vi "3D_Plotter_MATLAB.vi"(1 "Job Directory":path) -> (2 "Saved Automatically?":bool, 3 "gnuplotScript":string, 4 "Plot data file":path)   [LabVIEW 2022 SP3]
uses:
  Controls/Global_mode.ctl
  Data plotting/MATLAB/MATLAB_Mode.ctl
  <vilib>/Utility/error.llb/Trim Whitespace One-Sided.vi
  Results_plotter_Global.vi
  Globals/Constants_global.vi
  Data plotting/subVIs/Plot_Values_Global.vi
  <vilib>/Analysis/NI_AALBase.lvlib
panel:
  out "Output file":path
  out "Plot Folder":string[](array[string])
  out "Duplicate Plot":bool
  out "Selectors":i32[](array[numeric])
  out "stl filenames":string[][](array[string])
  out "Max Min array":dbl[][][][](array[numeric])
  out "stl Files":string[](array[string])
  out "stl Limits":sgl[][](array[numeric])
  out "C Limits":cluster{dbl[]}[](array[cluster])
  out "ldListDatafileShown":string[](array[string])
  out "Last Plot Index":i32[](array[numeric])
  out "Z per Figure":dbl[][](array[numeric])
  out "Y per Figure":dbl[][](array[numeric])
  out "X per Figure":dbl[][](array[numeric])
  out "All Z":dbl[](array[numeric])
  out "All Y":dbl[](array[numeric])
  out "All X":dbl[](array[numeric])
  out "Plot Titles":string[](array[string])
  out "Number of Figures":i32
  out "Plot":i32[][](array[numeric])
  out "X Labels":bool[](array[boolean])
  out "Y labels":bool[](array[boolean])
  in  "Tab Control":T1(tab)
  in  "Show Save Option?":bool
  in  "Font Size":string="10"
  in  "Height":string="0.02"
  in  "Width":string="0.2"
  in  "BottomEdge":string="0.05"
  in  "LeftEdge":string="0.4"
  in  "MainTitleFontSize":string="12"
  in  "Vectors":bool
  in  "Streamlines":bool
  in  "W Vector":u16(ring) items=["None", "Date of Measurement", "Time Measurement Commenced", "QA Code", "File", "Subproject", "Model Scale", "Hav (m)", "Spire Size", "Meas Instru Type", "Profile Type", "Ref Velocity (m/s)", "Uh_Uref Ratio", "Uref (m/s)", "Source Flow Rate (l/min)", "Stability", "Wind Direction (Deg)", "Wind Direction", "Magic Case", "Roughness Layout", "Turntable Size", "X (m) fs", "Y (m) fs", "Z (m) fs", "Z/Hav", "Legend1", "Legend2", "Legend3", "LegendDose", "Source", "X Pos (mm)", "Y Pos (mm)", "Z Pos (mm)", "Location XY fs", "U/Uref", "V/Uref", "W/Uref", "Wind speed/Uref", "u^2/Uref^2", "v^2/Uref^2", "w^2/Uref^2", "uv/Uref^2", "uw/Uref^2", "U (m/s)", "V (m/s)", "W (m/s)", "u^2 (m/s)^2", "v^2 (m/s)^2", "w^2 (m/s)^2", "uv (m/s)^2", "uw (m/s)^2", "U/Uref Std Error", "V/Uref Std Error", "W/Uref Std Error", "u^2/Uref^2 Std Error", "v^2/Uref^2 Std Error", "w^2/Uref^2 Std Error", "uv/Uref^2 Std Error", "uw/Uref^2 Std Error", "U (m/s) Std Error", "V (m/s) Std Error", "W (m/s) Std Error", "u^2 (m/s)^2 Std Error", "v^2 (m/s)^2 Std Error", "w^2 (m/s)^2 Std Error", "uv (m/s)^2 Std Error", "uw (m/s)^2 Std Error", "Atmos Pressure (mBar)", "Lab Ref Temperature (Deg C)", "Meas Time (min)", "Current Filepath", "Raw Data Filename", "Template File Used", "EnFlo_Tunnel Trav1 Pos Z", "EnFlo_Tunnel Trav1 Pos Y", "EnFlo_Tunnel Trav1 Pos X", "Coordinate System", "Original Results Filename", "Legend5", "Av LDA Sampling Rate", "Legend6", "Legend7", "K2", "Bldg12", "EnFlo_Tunnel Metadata Bldg12", "Current File 2nd Folder level"]
  in  "U Vector":u16(ring) items=["None", "Date of Measurement", "Time Measurement Commenced", "QA Code", "File", "Subproject", "Model Scale", "Hav (m)", "Spire Size", "Meas Instru Type", "Profile Type", "Ref Velocity (m/s)", "Uh_Uref Ratio", "Uref (m/s)", "Source Flow Rate (l/min)", "Stability", "Wind Direction (Deg)", "Wind Direction", "Magic Case", "Roughness Layout", "Turntable Size", "X (m) fs", "Y (m) fs", "Z (m) fs", "Z/Hav", "Legend1", "Legend2", "Legend3", "LegendDose", "Source", "X Pos (mm)", "Y Pos (mm)", "Z Pos (mm)", "Location XY fs", "U/Uref", "V/Uref", "W/Uref", "Wind speed/Uref", "u^2/Uref^2", "v^2/Uref^2", "w^2/Uref^2", "uv/Uref^2", "uw/Uref^2", "U (m/s)", "V (m/s)", "W (m/s)", "u^2 (m/s)^2", "v^2 (m/s)^2", "w^2 (m/s)^2", "uv (m/s)^2", "uw (m/s)^2", "U/Uref Std Error", "V/Uref Std Error", "W/Uref Std Error", "u^2/Uref^2 Std Error", "v^2/Uref^2 Std Error", "w^2/Uref^2 Std Error", "uv/Uref^2 Std Error", "uw/Uref^2 Std Error", "U (m/s) Std Error", "V (m/s) Std Error", "W (m/s) Std Error", "u^2 (m/s)^2 Std Error", "v^2 (m/s)^2 Std Error", "w^2 (m/s)^2 Std Error", "uv (m/s)^2 Std Error", "uw (m/s)^2 Std Error", "Atmos Pressure (mBar)", "Lab Ref Temperature (Deg C)", "Meas Time (min)", "Current Filepath", "Raw Data Filename", "Template File Used", "EnFlo_Tunnel Trav1 Pos Z", "EnFlo_Tunnel Trav1 Pos Y", "EnFlo_Tunnel Trav1 Pos X", "Coordinate System", "Original Results Filename", "Legend5", "Av LDA Sampling Rate", "Legend6", "Legend7", "K2", "Bldg12", "EnFlo_Tunnel Metadata Bldg12", "Current File 2nd Folder level"]
  in  "V Vector":u16(ring) items=["None", "Date of Measurement", "Time Measurement Commenced", "QA Code", "File", "Subproject", "Model Scale", "Hav (m)", "Spire Size", "Meas Instru Type", "Profile Type", "Ref Velocity (m/s)", "Uh_Uref Ratio", "Uref (m/s)", "Source Flow Rate (l/min)", "Stability", "Wind Direction (Deg)", "Wind Direction", "Magic Case", "Roughness Layout", "Turntable Size", "X (m) fs", "Y (m) fs", "Z (m) fs", "Z/Hav", "Legend1", "Legend2", "Legend3", "LegendDose", "Source", "X Pos (mm)", "Y Pos (mm)", "Z Pos (mm)", "Location XY fs", "U/Uref", "V/Uref", "W/Uref", "Wind speed/Uref", "u^2/Uref^2", "v^2/Uref^2", "w^2/Uref^2", "uv/Uref^2", "uw/Uref^2", "U (m/s)", "V (m/s)", "W (m/s)", "u^2 (m/s)^2", "v^2 (m/s)^2", "w^2 (m/s)^2", "uv (m/s)^2", "uw (m/s)^2", "U/Uref Std Error", "V/Uref Std Error", "W/Uref Std Error", "u^2/Uref^2 Std Error", "v^2/Uref^2 Std Error", "w^2/Uref^2 Std Error", "uv/Uref^2 Std Error", "uw/Uref^2 Std Error", "U (m/s) Std Error", "V (m/s) Std Error", "W (m/s) Std Error", "u^2 (m/s)^2 Std Error", "v^2 (m/s)^2 Std Error", "w^2 (m/s)^2 Std Error", "uv (m/s)^2 Std Error", "uw (m/s)^2 Std Error", "Atmos Pressure (mBar)", "Lab Ref Temperature (Deg C)", "Meas Time (min)", "Current Filepath", "Raw Data Filename", "Template File Used", "EnFlo_Tunnel Trav1 Pos Z", "EnFlo_Tunnel Trav1 Pos Y", "EnFlo_Tunnel Trav1 Pos X", "Coordinate System", "Original Results Filename", "Legend5", "Av LDA Sampling Rate", "Legend6", "Legend7", "K2", "Bldg12", "EnFlo_Tunnel Metadata Bldg12", "Current File 2nd Folder level"]
  in  "Manual_stl file":bool
  in  "Show whole Stl file":bool=TRUE
  in  "Stl File":u16(ring) items=["", "StreetCanyonGeometry.stl"]
  in  "Z Limits Auto":bool=TRUE
  in  "Location Z limits":string="-2000;2000"
  out "Y Limit":string
  out "X Limit":string
  in  "Concentration?":bool
  in  "Range Auto":bool=TRUE
  in  "Same Location limits for all plots":bool=TRUE
  in  "Swop Series and Plots":bool
  in  "mSingleColorbar":bool=TRUE
  in  "Y Limits Auto":bool=TRUE
  in  "X Limits Auto":bool=TRUE
  in  "Location X limits":string="-2000;2000"
  in  "nRows":u8=3 min=1
  in  "nCols":u8=3 min=1
  in  "cScatterPointSize":string="5"
  in  "Plotting":enum8{"Lin", "Log"}(ring)
  in  "fvectorRotation":string="0;0;0"
  in  "cdColorbarRange":string="0.01;100"
  in  "No Of decades":i32=3 min=1 max=10
  in  "Location Y limits":string="-2000;2000"
  out "Z Limit":string
  in  "ViewAngles":string="-115;35"
  in  "Transparency":string="0.5"
  in  "Streamline Density":string="0.5"
  in  "Open in Acrobat":bool=TRUE
  in  "Show Channels with range of Values?":bool
  in  "Page Title Pre Block":string
  in  "Page Title Post Block":string
  in  "Values to include in Page Title":i32[](listbox)
  out "Final Title":string
  out "Plot Legends Auto":string[](array[string])
  out "No of Series supplied":i32
  out "AuditTrail":string[](array[string])
  out "Desired Legends":string[][](array[string])
  out "Table":string[][](table)
  # "Plot XY axes control"
  # "Color Bar"
  # "Overall Page Title"
  # "There are as many graphs as there are titles (from Selector 2)...."
  # "Plot Styles"
  # "Each graph contains plots from Selector 1..."
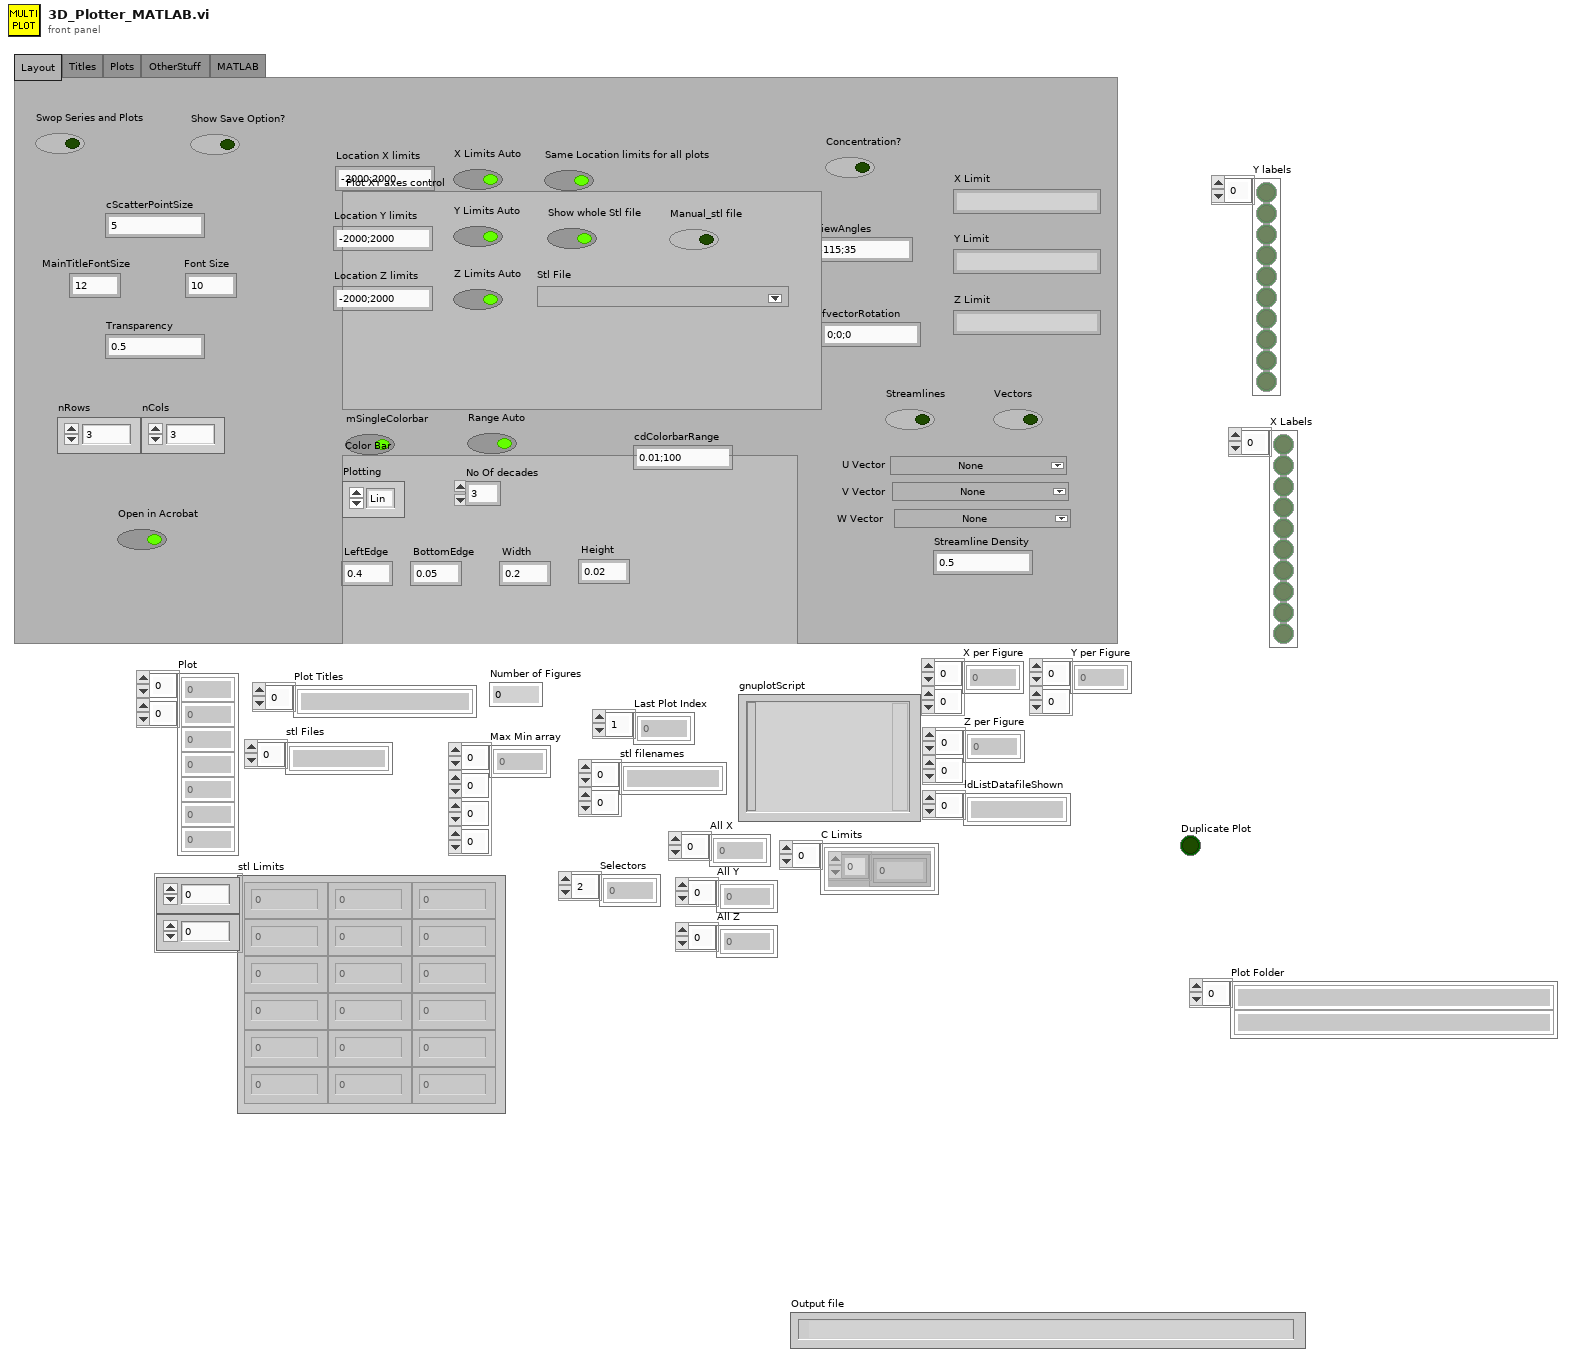
[diagram p1: front panel]
types:
  T1 = enum32{"Layout", "Titles", "Plots", "OtherStuff ", "MATLAB"}
  T2 = typedef "RFP_Plot_Metadata.ctl" = cluster{"Row Number":i32[], "Error Bars":T3, "X Label":string, "Y Label":string, "Blanks NaNs":i32[]}
  T3 = typedef "Error_bars_index.ctl" = cluster{"Upper":i32, "Lower":i32, "St Error":i32}
  T4 = typedef "Global_mode.ctl" = enum16{"Read Global", "Load Global From File", "Write Global to File"}
  T5 = typedef "MATLAB_Mode.ctl" = enum16{"1D Plotter", "2D Plotter", "LP Plotter", "7HP UVW"}
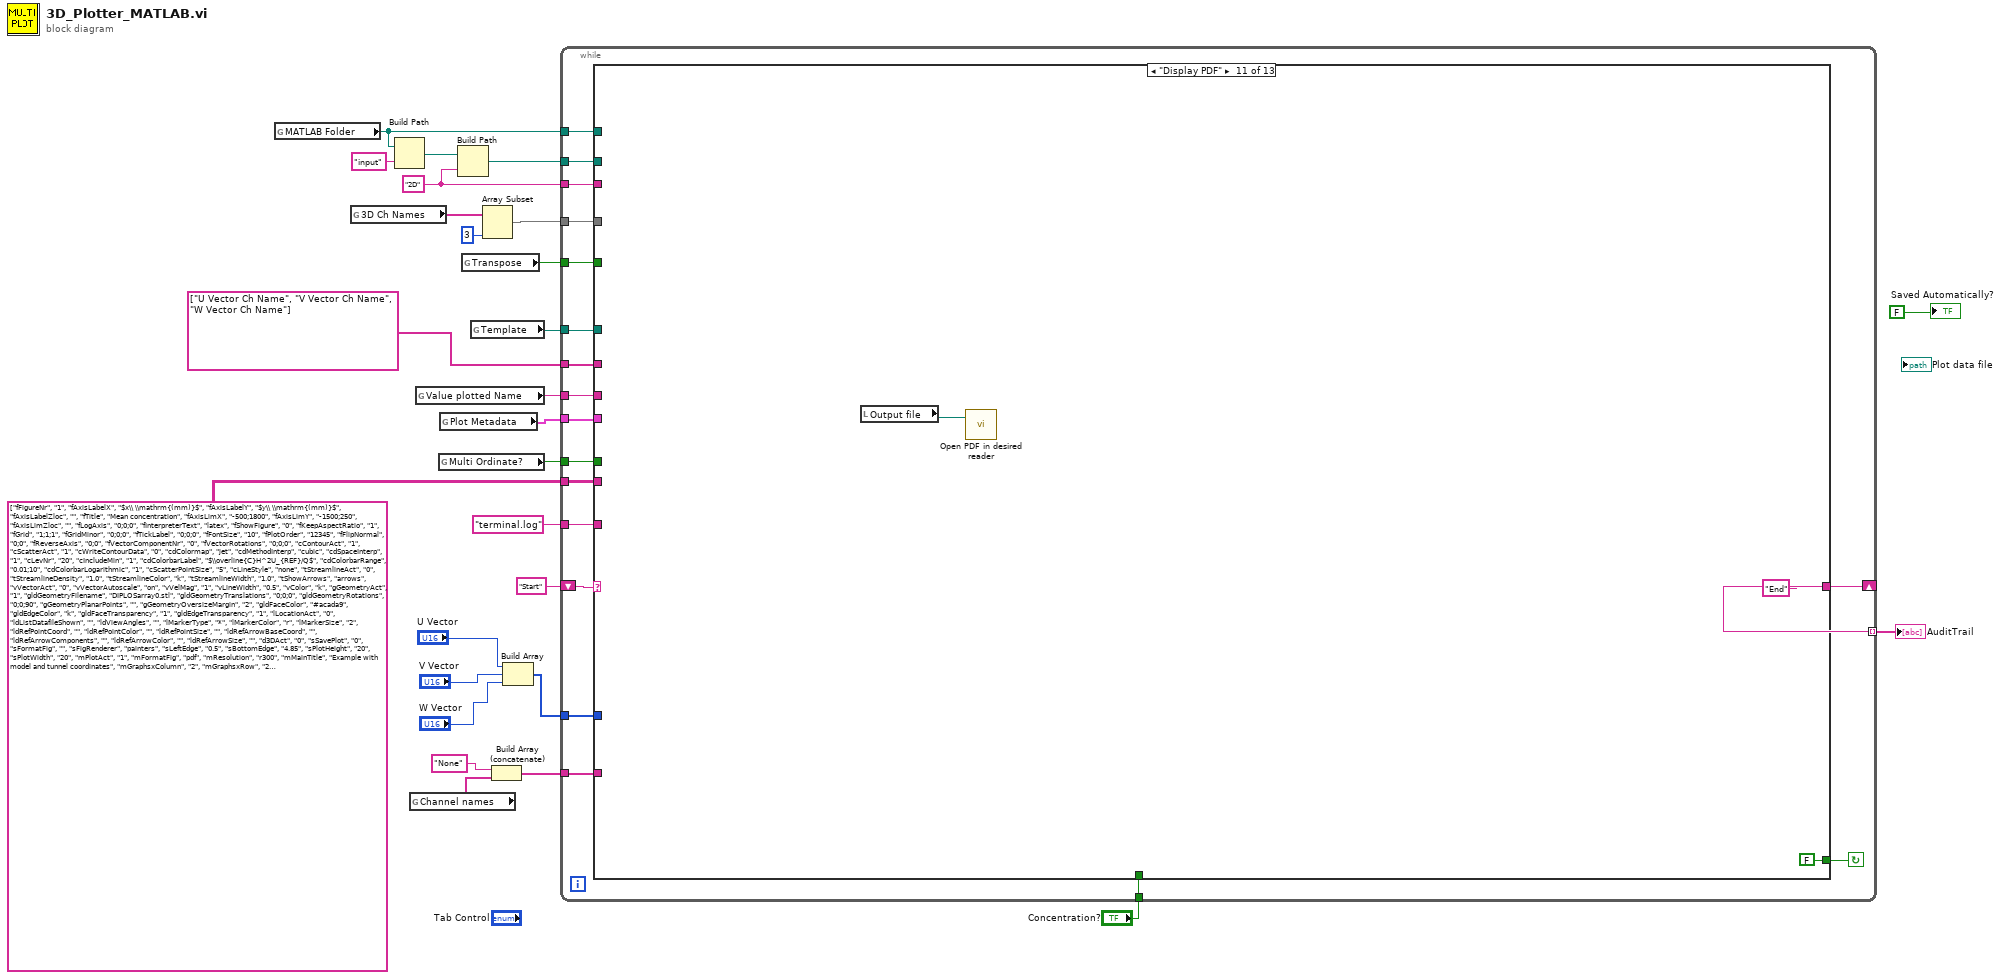
[diagram p0: block diagram]
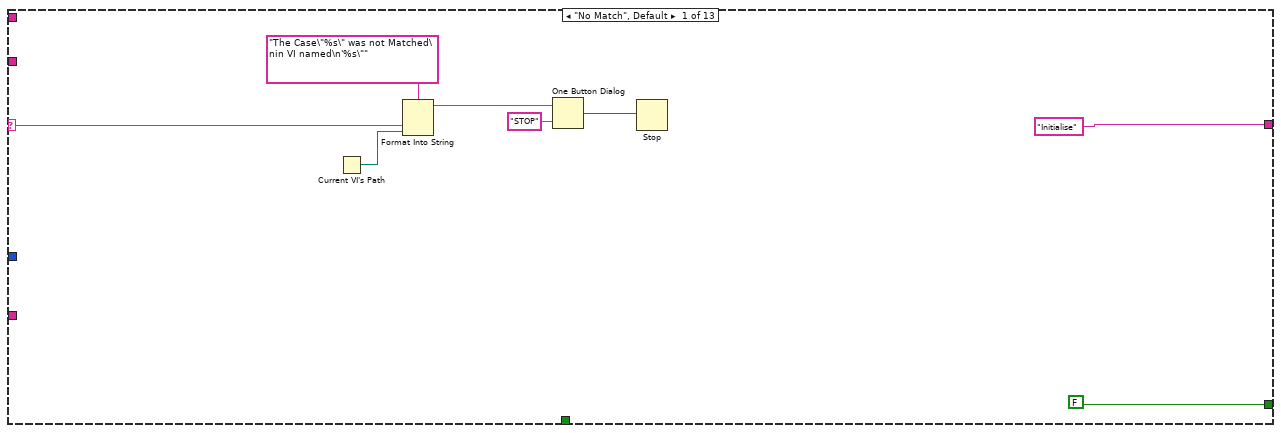
[diagram p2: hidden frame]
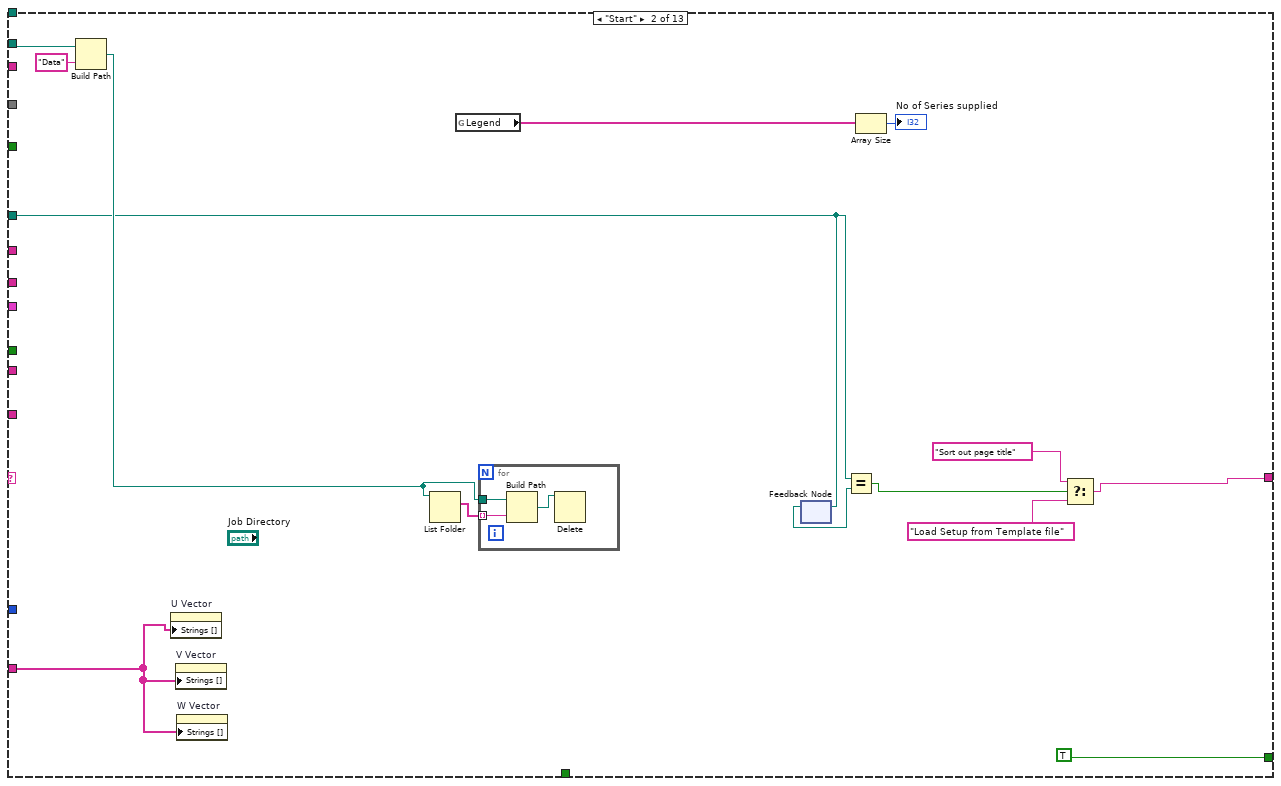
[diagram p3: hidden frame]
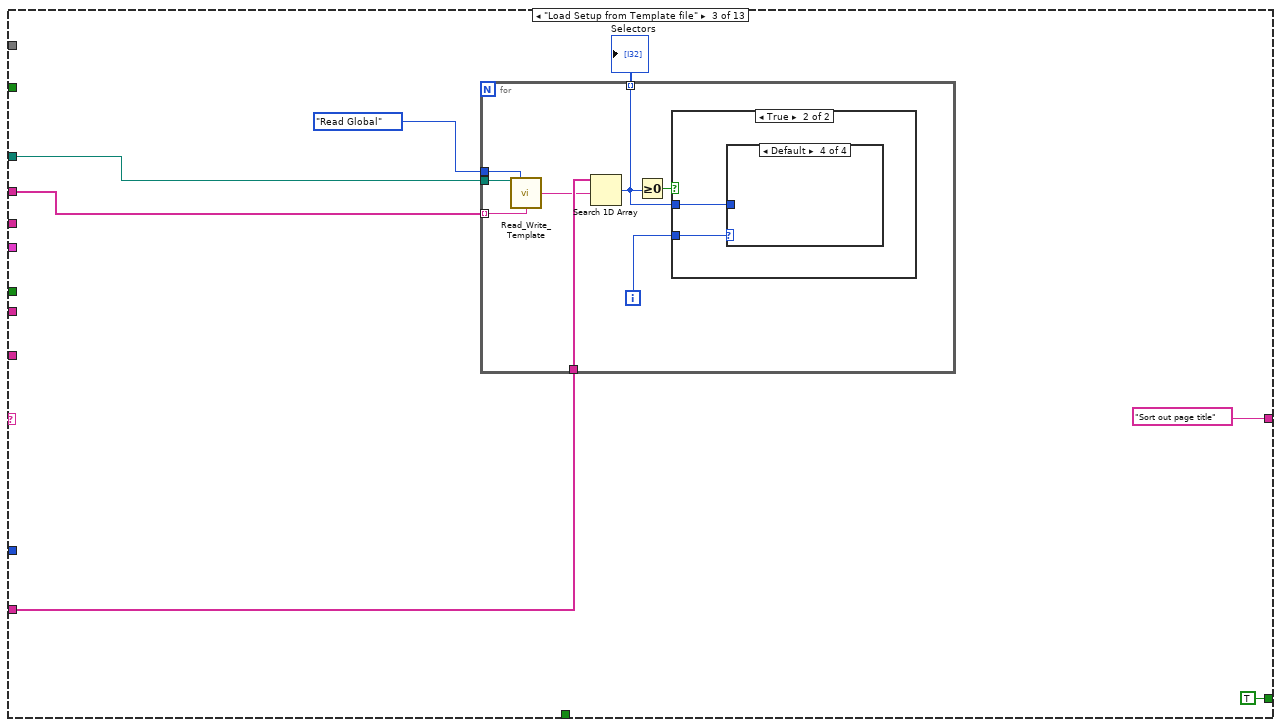
[diagram p4: hidden frame]
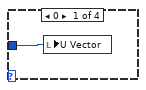
[diagram p6: hidden frame]
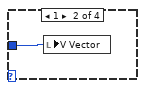
[diagram p7: hidden frame]
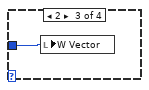
[diagram p8: hidden frame]
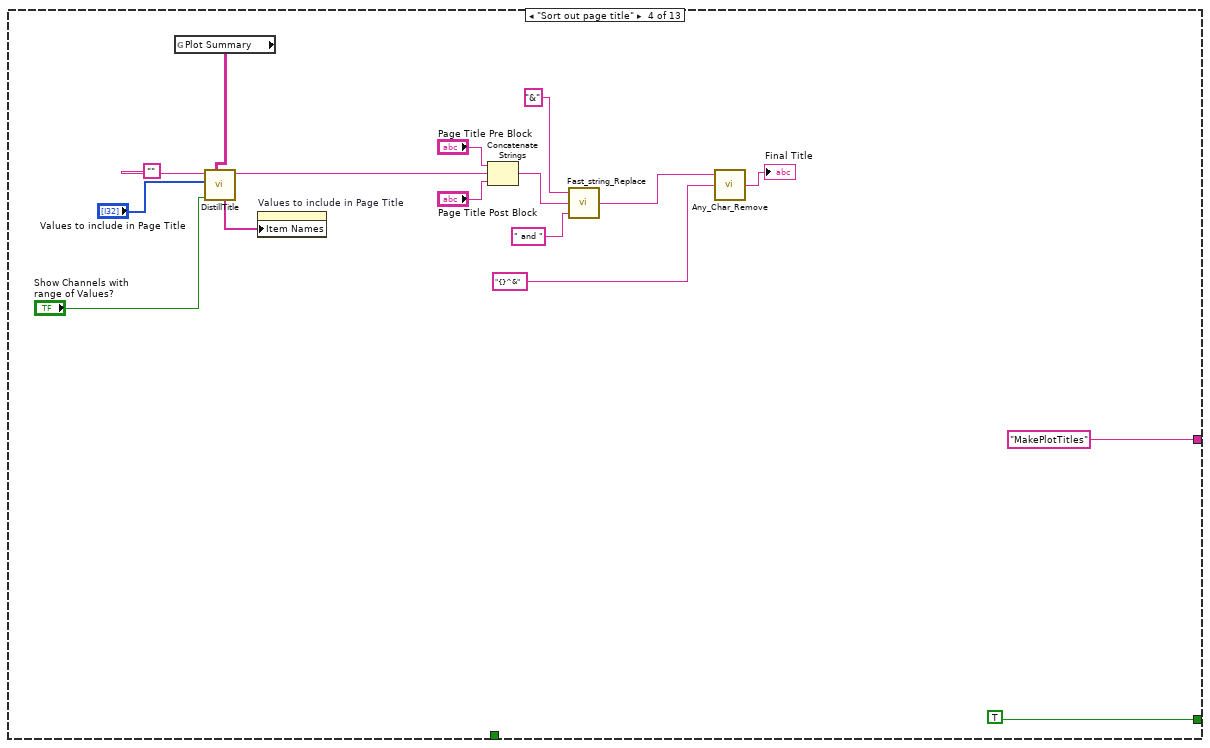
[diagram p9: hidden frame]
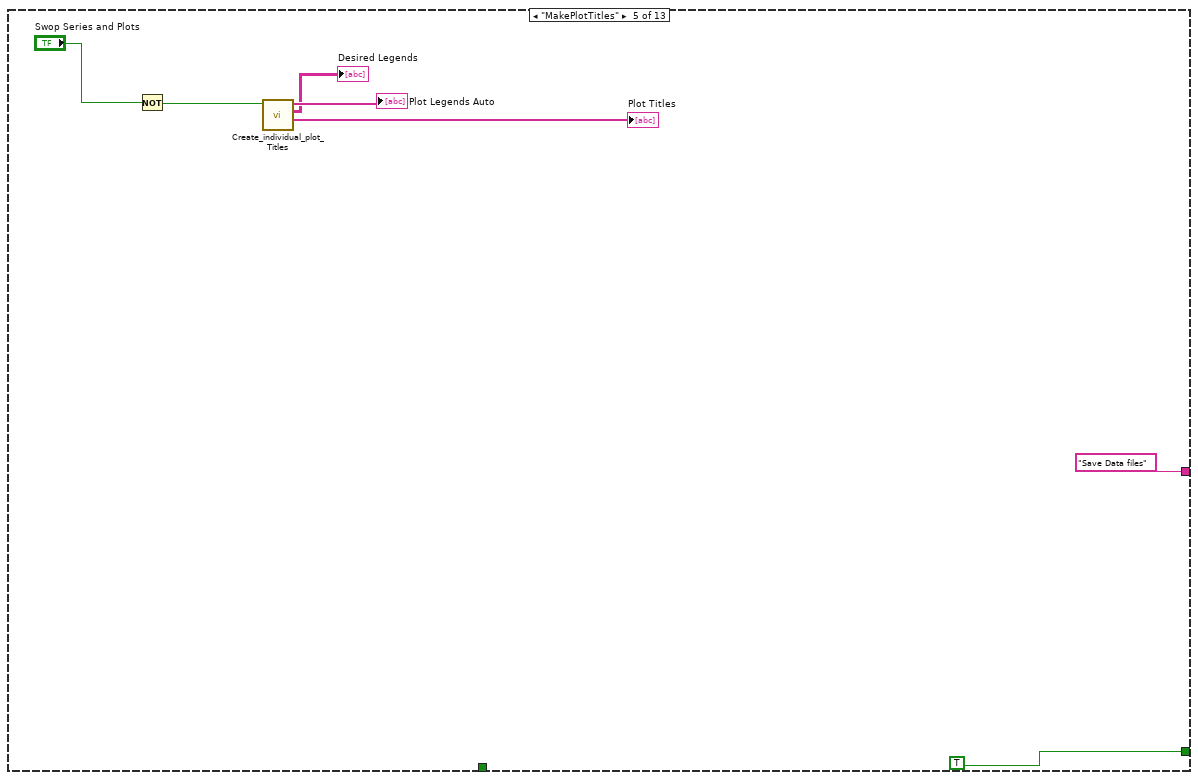
[diagram p10: hidden frame]
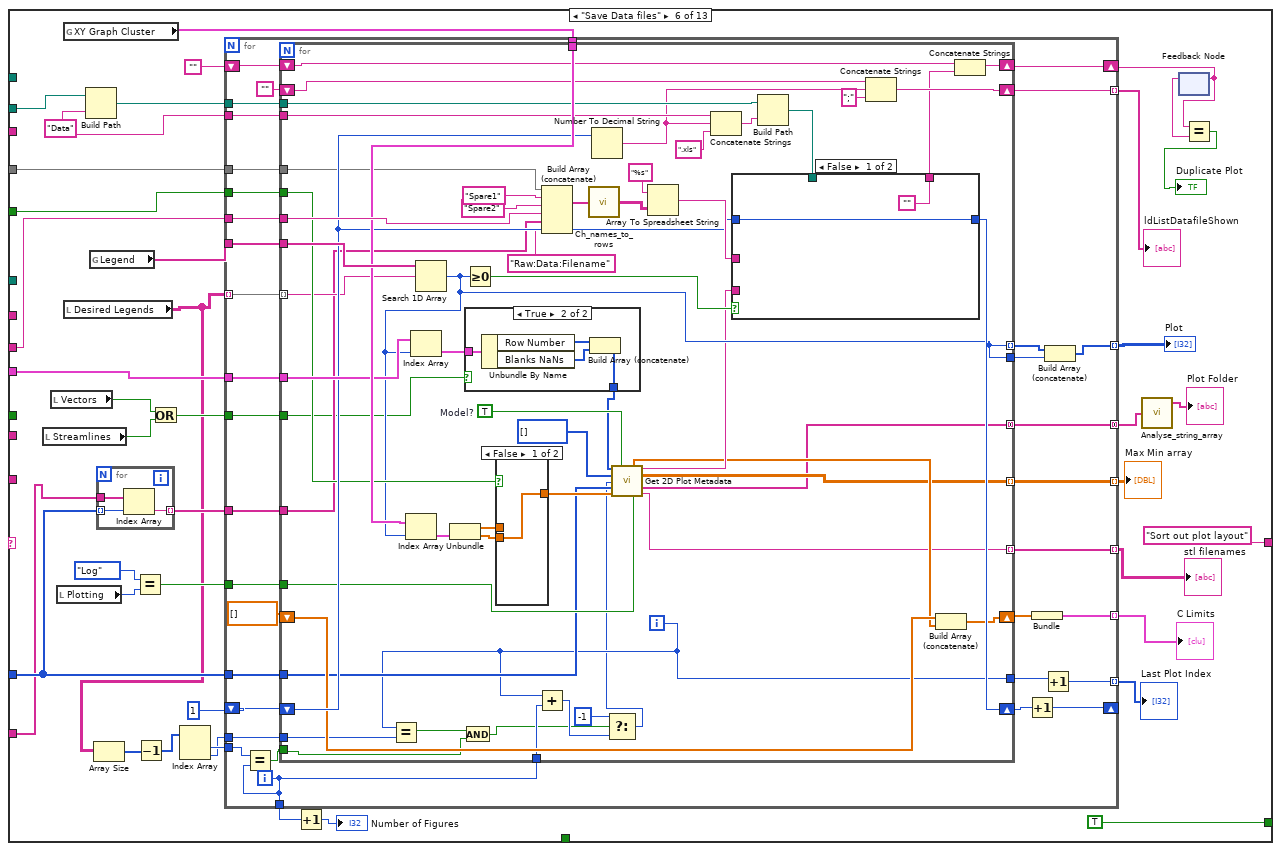
[diagram p11: hidden frame]
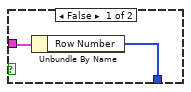
[diagram p12: hidden frame]
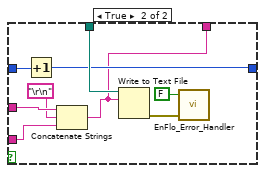
[diagram p14: hidden frame]
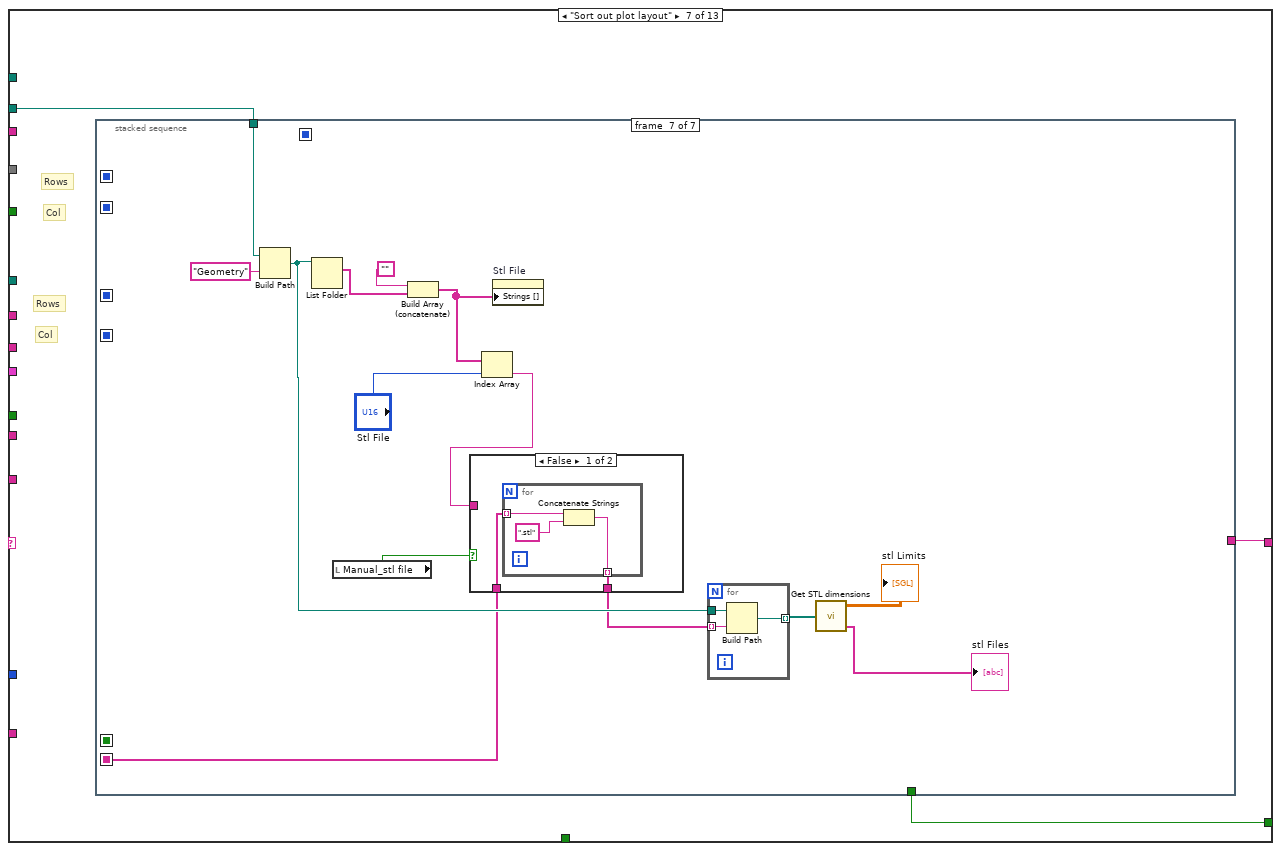
[diagram p15: hidden frame]
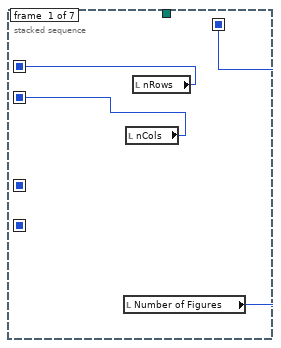
[diagram p16: hidden frame]
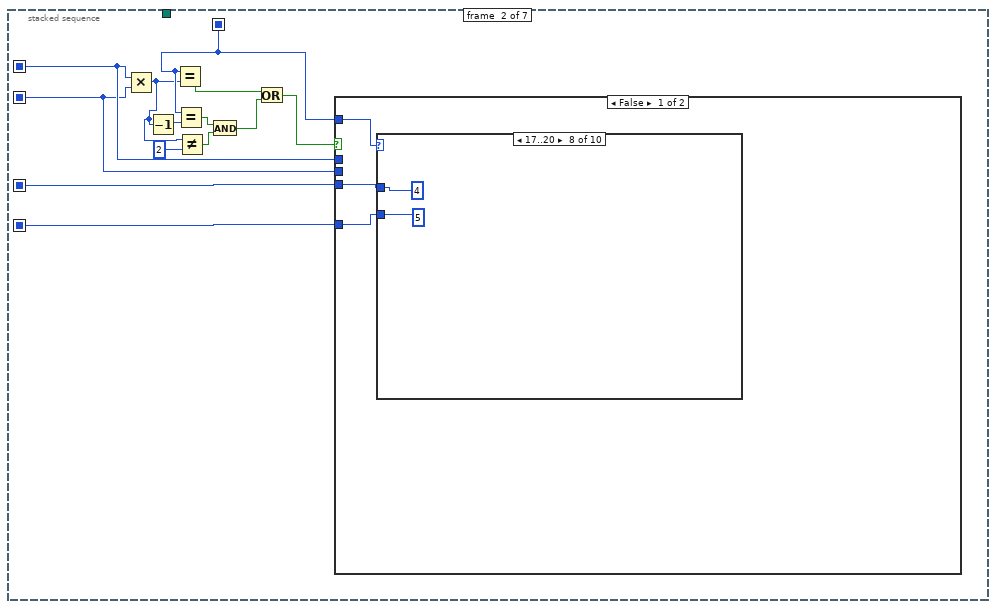
[diagram p17: hidden frame]
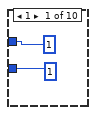
[diagram p18: hidden frame]
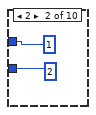
[diagram p19: hidden frame]
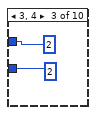
[diagram p20: hidden frame]
diagram:
  w1 = "2D" ("name or relative path")
  n1 = global read "Constants_global.vi" "MATLAB Folder"() -> (w2:path)
  n2 = global read "Results_plotter_Global.vi" "3D Ch Names"() -> (w13:string[])
  n3 = Build Path(base path=w2, name or relative path="input") -> (appended path=w19:path)
  n4 = global read "Results_plotter_Global.vi" "Channel names"() -> (w6:string[])
  n5 = global read "Results_plotter_Global.vi" "Value plotted Name"() -> (w26:string)
  n6 = global read "Results_plotter_Global.vi" "Multi Ordinate?"() -> (w22:bool)
  n7 = global read "Results_plotter_Global.vi" "Plot Metadata"() -> (w16:T2[])
  n8 = Build Path(base path=w19, name or relative path=w1) -> (appended path=w18:path)
  n9 = global read "Results_plotter_Global.vi" "Transpose"() -> (w23:bool)
  n10 = global read "Results_plotter_Global.vi" "Template"() -> (w4:path)
  n11 = Array Subset(array=w13, length=3) -> (w12:string[])  [unwired: 1 in]
  n12 = Build Array (concatenate)("None", w6) -> (w5:string[])
  n13 = Build Array("U Vector", "V Vector", "W Vector") -> (w8:u16[])
  n14 = while {
    shift-left: "Start" -> [w44]
    shift-right: [w39] -> _
    tunnel: w26 -> [w43]
    tunnel: "terminal.log" -> [w42]
    tunnel: w23 -> [w41]
    tunnel: w22 -> [w40]
    tunnel: [w39] -> w21 mode=indexing
    tunnel: w18 -> [w38]
    tunnel: string[][] [["fFigureNr", "1"], ["fAxisLabelX", "$x\\ \\mathrm{(mm)}$"], ["fAxisLabelY", "$y\\ \\mathrm{(mm)}$"], ["fAxisLabelZloc", ""], ["fTitle", "Mean concentration"], ["fAxisLimX", "-500;1800"], ["fAxisLimY", "-1500;250"], ["fAxisLimZloc", ""], ["fLogAxis", "0;0;0"], ["fInterpreterText", "latex"], ["fShowFigure", "0"], ["fKeepAspectRatio", "1"], ["fGrid", "1;1;1"], ["fGridMinor", "0;0;0"], ["fTickLabel", "0;0;0"], ["fFontSize", "10"], ["fPlotOrder", "12345"], ["fFlipNormal", "0;0"], ["fReverseAxis", "0;0"], ["fVectorComponentNr", "0"], ["fVectorRotations", "0;0;0"], ["cContourAct", "1"], ["cScatterAct", "1"], ["cWriteContourData", "0"], ["cdColormap", "jet"], ["cdMethodInterp", "cubic"], ["cdSpaceInterp", "1"], ["cLevNr", "20"], ["cIncludeMin", "1"], ["cdColorbarLabel", "$\\overline{C}H^2U_{REF}/Q$"], ["cdColorbarRange", "0.01;10"], ["cdColorbarLogarithmic", "1"], ["cScatterPointSize", "5"], ["cLineStyle", "none"], ["tStreamlineAct", "0"], ["tStreamlineDensity", "1.0"], ["tStreamlineColor", "k"], ["tStreamlineWidth", "1.0"], ["tShowArrows", "arrows"], ["vVectorAct", "0"], ["vVectorAutoscale", "on"], ["vVelMag", "1"], ["vLineWidth", "0.5"], ["vColor", "k"], ["gGeometryAct", "1"], ["gldGeometryFilename", "DIPLOSarray0.stl"], ["gldGeometryTranslations", "0;0;0"], ["gldGeometryRotations", "0;0;90"], ["gGeometryPlanarPoints", ""], ["gGeometryOversizeMargin", "2"], ["gldFaceColor", "#acada9"], ["gldEdgeColor", "k"], ["gldFaceTransparency", "1"], ["gldEdgeTransparency", "1"], ["lLocationAct", "0"], ["ldListDatafileShown", ""], ["ldViewAngles", ""], ["lMarkerType", "*"], ["lMarkerColor", "r"], ["lMarkerSize", "2"], ["ldRefPointCoord", ""], ["ldRefPointColor", ""], ["ldRefPointSize", ""], ["ldRefArrowBaseCoord", ""], ["ldRefArrowComponents", ""], ["ldRefArrowColor", ""], ["ldRefArrowSize", ""], ["d3DAct", "0"], ["sSavePlot", "0"], ["sFormatFig", ""], ["sFigRenderer", "painters"], ["sLeftEdge", "0.5"], ["sBottomEdge", "4.85"], ["sPlotHeight", "20"], ["sPlotWidth", "20"], ["mPlotAct", "1"], ["mFormatFig", "pdf"], ["mResolution", "r300"], ["mMainTitle", "Example with model and tunnel coordinates"], ["mGraphsxColumn", "2"], ["mGraphsxRow", "2"], ["mLeftEdge", "2"], ["mRightEdge", "1.5"], ["mTopEdge", "1.5"], ["mBottomEdge", "3"], ["mSpaceX", "2.2"], ["mSpaceY", "6"], ["mPlotHeight", "21"], ["mPlotWidth", "29.7"], ["mMainTitleFontSize", "12"], ["mFontSize", "10"], ["mInterpreterText", "latex"], ["mFigRenderer", "opengl"], ["mSingleColorbar", "0"], ["mSingleColorbarOrientation", "Horizontal"], ["mSingleColorbarLocation", "0.4;0.05;0.2;0.02"], ["dStreamlineSlice", "2"], ["dStreamlineStartPoint1", "0;0;0.5"], ["dStreamlineStartPoint2", "0;1;0.5"], ["dContourTransparency", "1"]] ("appended array") -> [w37]
    tunnel: w16 -> [w36]
    tunnel: "Concentration?" -> [w35]
    tunnel: w12 -> [w34]
    tunnel: w8 -> [w33]
    tunnel: w5 -> [w32]
    tunnel: w4 -> [w31]
    tunnel: string[] ["U Vector Ch Name", "V Vector Ch Name", "W Vector Ch Name"] -> [w30]
    tunnel: w2 -> [w29]
    tunnel: w1 -> [w28]
    stop <- w45 continue-if-true
    n15 = case shown="\"Display PDF\"" w44 {
      selector: w44 -> [w46 _ _ _ _ _ _ _ _ _ _ _ _]
      tunnel: [FALSE TRUE TRUE ("Top Level") TRUE ("Top Level") TRUE ("Top Level") TRUE ("Top Level") w271 TRUE ("Top Level") TRUE ("Top Level") w1049 FALSE ("Top Level") FALSE FALSE ("Top Level")] -> w45
      tunnel: ["Initialise" w57 "Sort out page title" "MakePlotTitles" "Save Data files" "Sort out plot layout" w269 "Save Input File" ("t") "Run MATLAB Code" ("t") w1044 "End" ("t") "" "End" ("t")] -> w39
      tunnel: w43 -> [_ _ _ _ _ w144 _ _ _ _ _ _ _]
      tunnel: w42 -> [_ _ _ _ _ _ _ _ _ _ _ _ _]
      tunnel: w41 -> [_ _ _ _ _ w153 _ _ _ _ _ _ _]
      tunnel: w40 -> [_ _ _ _ _ _ _ _ _ _ _ _ _]
      tunnel: w38 -> [_ w61 _ _ _ w148 w270 w507 w1018 _ _ _ _]
      tunnel: w37 -> [_ _ _ _ _ _ _ w514 _ _ _ _ _]
      tunnel: w36 -> [_ _ _ _ _ w138 _ _ _ _ _ _ _]
      tunnel: w35 -> [_ _ _ _ _ _ _ _ _ _ _ _ _]
      tunnel: w34 -> [_ _ _ _ _ w137 _ _ _ _ _ _ _]
      tunnel: w33 -> [_ _ _ _ _ w133 _ _ _ _ _ _ _]
      tunnel: w32 -> [_ w60 w74 _ _ w132 _ _ w1016 _ _ _ _]
      tunnel: w31 -> [_ w54 w76 _ _ _ _ _ w1017 _ _ _ _]
      tunnel: w30 -> [_ _ w75 _ _ _ _ _ w1014 _ _ _ _]
      tunnel: w29 -> [_ _ _ _ _ _ _ _ w1008 _ _ _ _]
      tunnel: w28 -> [_ _ _ _ _ _ _ _ w1007 _ _ _ _]
      frame "No Match", Default {
        n16 = Current VI's Path() -> (path=w48:path)
        n17 = Format Into String(format string="The Case\"%s\" was not Matched\nin VI named\n'%s\"" ("Format String"), w46, w48) -> (resulting string=w51:string)  [unwired: 2 in, 1 out]
        n18 = One Button Dialog(message=w51, button name ("OK")="STOP") -> (true=w49:bool)
        n19 = Stop(stop? (T)=w49) -> ()
      }
      frame "Start" {
        n20 = Build Path(base path=w61, name or relative path="Data") -> (appended path=w62:path)
        n21 = property on="U Vector" class="Ring (strict)"("Strings []"=w60) -> ()  [unwired: 2 in, 2 out]
        n22 = property on="V Vector" class="Ring (strict)"("Strings []"=w60) -> ()  [unwired: 2 in, 2 out]
        n23 = property on="W Vector" class="Ring (strict)"("Strings []"=w60) -> ()  [unwired: 2 in, 2 out]
        n24 = List Folder(path=w62) -> (filenames=w64:string[])  [unwired: 3 in, 3 out]
        n25 = global read "Results_plotter_Global.vi" "Legend"() -> (w65:string[])
        n26 = for {
          tunnel: w64 -> [w70] mode=indexing
          tunnel: w62 -> [w69]
          n27 = Build Path(base path=w69, name or relative path=w70) -> (appended path=w68:path)
          n28 = Delete(path (use dialog)=w68) -> ()  [unwired: 4 in, 3 out]
        }
        n29 = feedback-in #1(w54) -> ()
        n30 = feedback #1() -> (w59:path)  [unwired: 1 in]
        n31 = Equal?(x=w54, y=w59) -> (x = y?=w55:bool)
        n32 = Array Size(array=w65) -> (size(s)=→"No of Series supplied":i32)
        n33 = Select(t="Sort out page title", s=w55, f="Load Setup from Template file") -> (s? t:f=w57:string)
      }
      frame "Load Setup from Template file" {
        n34 = for {
          tunnel: w76 -> [w85]
          tunnel: Global_mode."Read Global" ("Mode") -> [w84]
          tunnel: w75 -> [w83] mode=indexing
          tunnel: w74 -> [w82]
          tunnel: [w78] -> w73 mode=indexing
          i -> [w80]
          n35 = call "Read_Write_Template.vi"("Template File"=w85, "Mode"=w84, "Data type"=w83) -> ("Single Value Out"=w81:string)  [unwired: 5 in, 7 out]
          n36 = Search 1D Array(1D array=w82, element=w81) -> (index of element=w78:i32)  [unwired: 1 in]
          n37 = Greater Or Equal To 0?(x=w78) -> (x >= 0?=w79:bool)
          n38 = case shown="True" w79 {
            tunnel: w80 -> [_ w87]
            tunnel: w78 -> [_ w86]
            frame False {
            }
            frame True {
              n39 = case shown="Default" w87 {
                tunnel: w86 -> [w88 w89 w90 _]
                frame 0 {
                  n40 = local write "U Vector"(w88) -> ()
                }
                frame 1 {
                  n41 = local write "V Vector"(w89) -> ()
                }
                frame 2 {
                  n42 = local write "W Vector"(w90) -> ()
                }
                frame Default {
                }
              }
            }
          }
        }
        "Selectors" <- w73
      }
      frame "Sort out page title" {
        n43 = global read "Results_plotter_Global.vi" "Plot Summary"() -> (w92:string[][])
        n44 = call "DistillTitle.vi"("Plot Summary in"=w92, "Show Channels with range of Values?"="Show Channels with range of Values?", "Indices to include in Page Title"="Values to include in Page Title", "String in"="") -> ("String out"=w105:string, "AvailableVariables"=w100:string[])  [unwired: 6 in]
        n45 = property on="Values to include in Page Title" class="LstBox (strict)"("Item Names"=w100) -> ()  [unwired: 2 in, 2 out]
        n46 = Concatenate Strings("Page Title Pre Block", w105, "Page Title Post Block") -> (w96:string)
        n47 = call "Fast_string_Replace.vi"("Replace match with:"=" and " ("Individual Characters to Remove"), "Input String"=w96, "matchThis"="&" ("Individual Characters to Remove")) -> ("Output String"=w93:string)  [unwired: 1 in, 1 out]
        n48 = call "Any_Char_Remove.vi"("Individual Characters to Remove"="{}^&", "String in"=w93) -> ("String out"=→"Final Title":string)  [unwired: 1 in]
      }
      frame "MakePlotTitles" {
        n49 = Not(x="Swop Series and Plots") -> (.not. x?=w107:bool)
        n50 = call "Create_individual_plot_Titles.vi"("Swop Series and Plots"=w107) -> ("1D Plot Titles"=→"Plot Titles":string[], "Desired Legends"=→"Desired Legends":string[][], "Plot Legends Auto"=→"Plot Legends Auto":string[])  [unwired: 2 in, 2 out]
      }
      frame "Save Data files" {
        w147 = "Data" ("name or relative path")
        n51 = local read "Streamlines"() -> (w121:bool)
        n52 = local read "Vectors"() -> (w120:bool)
        n53 = local read "Plotting"() -> (w136:enum8{"Lin", "Log"})
        n54 = global read "Plot_Values_Global.vi" "XY Graph Cluster"() -> (w128:cluster{dbl[], dbl[]}[])
        n55 = local read "Desired Legends"() -> (w118:string[][])
        n56 = Build Path(base path=w148, name or relative path=w147) -> (appended path=w146:path)
        n57 = global read "Results_plotter_Global.vi" "Legend"() -> (w149:string[])
        n58 = Array Size(array=w118) -> (size(s)=w117:i32[])
        n59 = for {
          tunnel: w133 -> [w156] mode=indexing
          tunnel: w132 -> [w155]
          tunnel: [w154] -> w131 mode=indexing
          n60 = Index Array(array=w155, index=w156) -> (element=w154:string)
        }
        n61 = Equal?(x=enum8{"Lin", "Log"}."Log" ("Plotting"), y=w136) -> (x = y?=w134:bool)
        n62 = Decrement(x=w117) -> (x-1=w116:i32[])
        n63 = Or(x=w120, y=w121) -> (x .or. y?=w119:bool)
        n64 = Index Array(array=w116) -> (element #1=w115:i32, element #2=w114:i32)  [unwired: 2 in]
        n65 = for {
          tunnel: w153 -> [w191]
          tunnel: w128 -> [w190]
          tunnel: w149 -> [w189]
          tunnel: w138 -> [w188]
          tunnel: w147 -> [w187]
          tunnel: w146 -> [w186]
          tunnel: [w182] -> w145 mode=indexing
          tunnel: w144 -> [w185]
          shift-right: [w181] -> _
          shift-left: 1 -> [w161]
          tunnel: w118 -> [w184] mode=indexing
          tunnel: [w157] -> w142
          tunnel: [w178] -> w141 mode=indexing
          tunnel: [w176] -> w140 mode=indexing
          tunnel: [w173] -> w139 mode=indexing
          tunnel: w137 -> [w171]
          tunnel: w134 -> [w170]
          tunnel: w133 -> [w169]
          tunnel: w131 -> [w168]
          tunnel: [w167] -> w130 mode=indexing
          tunnel: [w166] -> w129 mode=indexing
          tunnel: [w165] -> w127 mode=concatenating
          shift-right: [w163] -> w123
          shift-left: "" -> [w164]
          tunnel: w119 -> [w162]
          tunnel: w115 -> [w160]
          tunnel: w114 -> [w159]
          i -> [w157]
          n66 = Equal?(x=w160, y=w157) -> (x = y?=w158:bool)
          n67 = for {
            tunnel: w191 -> [w231]
            tunnel: w190 -> [w242]
            shift-right: [w232] -> w180
            shift-left: w161 -> [w233]
            tunnel: w185 -> [w247]
            tunnel: w189 -> [w243]
            tunnel: w184 -> [w228] mode=indexing
            tunnel: w188 -> [w240]
            tunnel: w187 -> [w237]
            tunnel: w186 -> [w235]
            tunnel: [w226] -> w172 mode=indexing
            tunnel: [w226] -> w183
            tunnel: [w196] -> w179
            shift-right: [w223] -> w176
            shift-left: "" -> [w222]
            shift-right: [w220] -> w174
            shift-left: dbl[] [] -> [w221]
            tunnel: w171 -> [w218]
            tunnel: w170 -> [w216]
            tunnel: w169 -> [w212]
            tunnel: w168 -> [w211]
            tunnel: [w210] -> w167 mode=indexing
            tunnel: [w209] -> w166 mode=indexing
            tunnel: [w207] -> w165 mode=concatenating
            shift-right: [w204] -> w163
            shift-left: w164 -> [w205]
            tunnel: w162 -> [w202]
            tunnel: w159 -> [w200]
            tunnel: w158 -> [w198]
            tunnel: w157 -> [w197]
            i -> [w196]
            w215 = TRUE  # Model?
            n68 = Equal?(x=w196, y=w200) -> (x = y?=w199:bool)
            n69 = Search 1D Array(1D array=w243, element=w228) -> (index of element=w226:i32)  [unwired: 1 in]
            n70 = Index Array(array=w242, index=w226) -> (element=w241:cluster{dbl[], dbl[]})
            n71 = Index Array(array=w240, index=w226) -> (element=w203:T2)
            n72 = Unbundle(w241) -> (w230:dbl[], w229:dbl[])
            n73 = And(x=w199, y=w198) -> (x .and. y?=w194:bool)
            n74 = Greater Or Equal To 0?(x=w226) -> (x >= 0?=w227:bool)
            n75 = case shown="True" w202 {
              tunnel: w203 -> [w251 w255]
              tunnel: [w250 w252] -> w201
              frame False {
                n76 = Unbundle By Name(w251) -> ("Row Number"=w250:i32[])
              }
              frame True {
                n77 = Unbundle By Name(w255) -> ("Row Number"=w254:i32[], "Blanks NaNs"=w253:i32[])
                n78 = Build Array (concatenate)(w254, w253) -> (w252:i32[])
              }
            }
            n79 = case shown="False" w231 {
              tunnel: [w256 w257] -> w217
              tunnel: w230 -> [_ w257]
              tunnel: w229 -> [w256 _]
              frame False {
              }
              frame True {
              }
            }
            n80 = Add(x=w196, y=w197) -> (x+y=w195:i32)
            n81 = Build Array (concatenate)(w218, "Spare1", "Spare2", w247, w211, "Raw:Data:Filename" ("element")) -> (w244:string[])
            n82 = call "Ch_names_to_rows.vi"("Channel Names"=w244) -> ("3 Row names"=w246:string[][])
            n83 = Number To Decimal String(number=w233) -> (decimal integer string=w225:string)  [unwired: 1 in]
            n84 = Select(t=-1, s=w194, f=w195) -> (s? t:f=w192:i32)
            n85 = call "Get 2D Plot Metadata.vi"("Row Number"=w201, "Model?"=w215, "Source Location"=i32[] [], "Interation number"=w192, "UVW index"=w212, "Scalar Value"=w217, "Log Plot?"=w216) -> ("Scalar limits"=w213:dbl[], "spreadsheet string"=w214:string, "Max Min array"=w210:dbl[][], "Data Directories"=w207:string[], "Stl Filename"=w209:string)  [unwired: 2 in, 2 out]
            n86 = Array To Spreadsheet String(array=w246, 3:"%s" ("format string")) -> (spreadsheet string=w239:string)  [unwired: 1 out]
            n87 = Concatenate Strings(w237, w225, ".xls" ("string")) -> (w236:string)
            n88 = Build Path(base path=w235, name or relative path=w236) -> (appended path=w234:path)
            n89 = case shown="False" w227 {
              tunnel: w234 -> [_ w268]
              tunnel: w239 -> [_ w267]
              tunnel: w214 -> [_ w262]
              tunnel: [w259 w263] -> w232
              tunnel: w233 -> [w259 w264]
              tunnel: ["" w260] -> w206
              frame False {
              }
              frame True {
                n90 = Increment(x=w264) -> (x+1=w263:i32)
                n91 = Concatenate Strings(w267, "\r\n", w262) -> (w260:string)
                n92 = Write to Text File(file (use dialog)=w268, text=w260) -> (error out=w266:errorcluster)  [unwired: 2 in, 2 out]
                n93 = call "EnFlo_Error_Handler.vi"("error in (no error)"=w266, "Dialog Box (F)"=FALSE ("Dialog Box (T)")) -> ()  [unwired: 2 in, 2 out]
              }
            }
            n94 = Concatenate Strings(w222, w225, ";" ("string")) -> (w223:string)
            n95 = Build Array (concatenate)(w221, w213) -> (w220:dbl[])
            n96 = Concatenate Strings(w205, w206) -> (w204:string)
          }
          n97 = Increment(x=w180) -> (x+1=w181:i32)
          n98 = Bundle(w174) -> (w173:cluster{dbl[]})  [unwired: 1 in]
          n99 = Increment(x=w179) -> (x+1=w178:i32)
          n100 = Build Array (concatenate)(w172, w183) -> (w182:i32[])
        }
        "Plot" <- w145
        "Last Plot Index" <- w141
        "ldListDatafileShown" <- w140
        "C Limits" <- w139
        "Max Min array" <- w130
        "stl filenames" <- w129
        n101 = Increment(x=w142) -> (x+1=→"Number of Figures":i32)
        n102 = call "Analyse_string_array.vi"("String array"=w127) -> ("Unique strings"=→"Plot Folder":string[])  [unwired: 1 in, 1 out]
        n103 = feedback #2() -> (w124:string)  [unwired: 1 in]
        n104 = feedback-in #2(w123) -> ()
        n105 = Equal?(x=w123, y=w124) -> (x = y?=→"Duplicate Plot":bool)
      }
      frame "Sort out plot layout" {
        # "Col"
        # "Rows"
        # "Col"
        # "Rows"
        n106 = stacked-sequence {
          seq-local: [w274 _ _ _ _ _ _] -> [_ w286 _ _ _ _ _]
          seq-local: [w273 _ _ _ _ _ _] -> [_ w284 _ _ _ _ _]
          seq-local: [_ w287 _ _ _ _ _] -> [_ _ w317 w354 _ _ _]
          seq-local: [_ w285 _ _ _ _ _] -> [_ _ w318 w353 _ _ _]
          seq-local: [w272 _ _ _ _ _ _] -> [_ w282 w313 w351 _ _ _]
          seq-local: [_ _ _ _ w375 _ _] -> [_ _ _ _ _ w478 _]
          seq-local: [_ _ _ _ w358 _ _] -> [_ _ _ _ _ _ w483]
          tunnel: [_ _ _ _ _ w476 _] -> w271
          tunnel: w270 -> [_ _ _ _ _ _ w484]
          tunnel: [_ _ _ _ "Create Input file" _ _] -> w269
          frame #0 {
            n107 = local read "Number of Figures"() -> (w272:i32)
            n108 = local read "nCols"() -> (w273:u8)
            n109 = local read "nRows"() -> (w274:u8)
          }
          frame #1 {
            n110 = Multiply(x=w286, y=w284) -> (x*y=w279:u8)
            n111 = Decrement(x=w279) -> (x-1=w283:u8)
            n112 = Equal?(x=w282, y=w279) -> (x = y?=w281:bool)
            n113 = Equal?(x=w282, y=w283) -> (x = y?=w276:bool)
            n114 = Not Equal?(x=w279, y=u8 2) -> (x != y?=w277:bool)
            n115 = And(x=w276, y=w277) -> (x .and. y?=w275:bool)
            n116 = Or(x=w281, y=w275) -> (x .or. y?=w280:bool)
            n117 = case shown="False" w280 {
              tunnel: w282 -> [w288 _]
              tunnel: [w290 w312] -> w287
              tunnel: w286 -> [_ w312]
              tunnel: [w289 w311] -> w285
              tunnel: w284 -> [_ w311]
              frame False {
                n118 = case shown="17..20" w288 {
                  tunnel: [u8 1 ("nRows") u8 2 ("nRows") u8 2 ("nRows") u8 3 ("nRows") u8 3 ("nRows") u8 4 ("nRows") u8 4 ("nRows") u8 5 ("nRows") u8 5 ("nRows") u8 6 ("nRows")] -> w289
                  tunnel: [u8 1 ("nRows") u8 1 ("nRows") u8 2 ("nRows") u8 2 ("nRows") u8 3 ("nRows") u8 3 ("nRows") u8 4 ("nRows") u8 4 ("nRows") u8 5 ("nRows") u8 5 ("nRows")] -> w290
                  frame 1 {
                  }
                  frame 2 {
                  }
                  frame 3, 4 {
                  }
                  frame 5, 6 {
                  }
                  frame 7..9 {
                  }
                  frame 10..12 {
                  }
                  frame 13..16 {
                  }
                  frame 17..20 {
                  }
                  frame 21..25 {
                  }
                  frame 26, Default {
                  }
                }
              }
              frame True {
              }
            }
          }
          frame #2 {
            n119 = local write "nRows"(w317) -> ()
            n120 = local write "nCols"(w318) -> ()
            n121 = for {
              N: w317 -> [_]
              tunnel: w318 -> [w341]
              tunnel: w313 -> [w340]
              tunnel: [w339] -> w319 mode=indexing
              tunnel: [w337] -> w320 mode=concatenating
              i -> [w342]
              n122 = Multiply(x=w341, y=w342) -> (x*y=w338:i32)
              n123 = for {
                N: w341 -> [_]
                tunnel: w338 -> [w350]
                tunnel: w340 -> [w349]
                tunnel: [w343] -> w339 mode=indexing
                tunnel: [w347] -> w337 mode=indexing
                i -> [w348]
                n124 = Add(x=w350, y=w348) -> (x+y=w345:i32)
                n125 = Equal To 0?(x=w348) -> (x = 0?=w347:bool)
                n126 = Less?(x=w345, y=w349) -> (x < y?=w346:bool)
                n127 = Select(t=w345, s=w346, f=-1) -> (s? t:f=w343:i32)
              }
            }
            "Y labels" <- w320
            n128 = Decrement(x=w317) -> (x-1=w316:u8)
            n129 = for {
              N: w318 -> [_]
              tunnel: w319 -> [w327]
              tunnel: w316 -> [w329]
              tunnel: [w326] -> w315 mode=indexing
              i -> [w330]
              n130 = Index Array(array=w327, index (row)=w329, index (col)=w330) -> (element=w325:i32)
              n131 = Decrement(x=w329) -> (x-1=w328:u8)
              n132 = Less Than 0?(x=w325) -> (x < 0?=w331:bool)
              n133 = case shown="False" w331 {
                tunnel: w330 -> [_ w336]
                tunnel: w328 -> [_ w335]
                tunnel: w327 -> [_ w334]
                tunnel: [w332 w333] -> w326
                tunnel: w325 -> [w332 _]
                frame False {
                }
                frame True {
                  n134 = Index Array(array=w334, index (row)=w335, index (col)=w336) -> (element=w333:i32)
                }
              }
            }
            n135 = for {
              N: w313 -> [_]
              tunnel: w315 -> [w324]
              tunnel: [w321] -> w314 mode=indexing
              i -> [w323]
              n136 = Search 1D Array(1D array=w324, element=w323) -> (index of element=w322:i32)  [unwired: 1 in]
              n137 = Greater Or Equal To 0?(x=w322) -> (x >= 0?=w321:bool)
            }
            "X Labels" <- w314
          }
          frame #3 {
            n138 = Multiply(x=w354, y=w353) -> (x*y=w352:u8)
            n139 = Equal?(x=w351, y=w352) -> ()  [unwired: 1 out]
          }
          frame #4 {
            w374 = dbl[] []
            n140 = local read "Max Min array"() -> (w356:dbl[][][][])
            n141 = local read "stl filenames"() -> (w355:string[][])
            n142 = for {
              tunnel: [w404] -> w375
              shift-right: [w397] -> w373
              shift-left: w374 -> [w403]
              shift-right: [w398] -> w363
              shift-left: w374 -> [w402]
              shift-right: [w399] -> w362
              shift-left: w374 -> [w401]
              tunnel: w374 -> [w400]
              tunnel: [w387] -> w361 mode=indexing
              tunnel: [w386] -> w360 mode=indexing
              tunnel: [w385] -> w359 mode=indexing
              tunnel: [w383] -> w358 mode=indexing
              tunnel: w356 -> [w382] mode=indexing
              tunnel: w355 -> [w381] mode=indexing
              n143 = for {
                shift-right: [w427] -> w397
                shift-left: w403 -> [w428]
                shift-right: [w424] -> w398
                shift-left: w402 -> [w426]
                shift-right: [w423] -> w399
                shift-left: w401 -> [w425]
                tunnel: [w416] -> w404 mode=indexing
                shift-right: [w412] -> w390
                shift-left: w400 -> [w415]
                shift-right: [w411] -> w389
                shift-left: w400 -> [w414]
                shift-right: [w410] -> w388
                shift-left: w400 -> [w413]
                tunnel: [w408] -> w384 mode=indexing
                tunnel: w382 -> [w409] mode=indexing
                tunnel: w381 -> [w408] mode=indexing
                n144 = for {
                  tunnel: w409 -> [w430] mode=indexing
                  tunnel: [w445] -> w421 mode=indexing
                  shift-right: [w442] -> w427
                  shift-left: w428 -> [w443]
                  shift-right: [w441] -> w424
                  shift-left: w426 -> [w440]
                  shift-right: [w439] -> w423
                  shift-left: w425 -> [w438]
                  shift-right: [w433] -> w412
                  shift-left: w415 -> [w434]
                  shift-right: [w432] -> w411
                  shift-left: w414 -> [w435]
                  shift-right: [w436] -> w410
                  shift-left: w413 -> [w437]
                  i -> [w431]
                  n145 = case shown="0, Default" w431 {
                    tunnel: w443 -> [w465 w470 w475]
                    tunnel: w430 -> [w464 w468 w473]
                    tunnel: [w463 w470 w475] -> w442
                    tunnel: [w462 w467 w471] -> w441
                    tunnel: w440 -> [w462 w469 w471]
                    tunnel: [w461 w466 w472] -> w439
                    tunnel: w438 -> [w461 w466 w474]
                    frame 0, Default {
                      n146 = Build Array (concatenate)(w465, w464) -> (w463:dbl[])
                    }
                    frame 1 {
                      n147 = Build Array (concatenate)(w469, w468) -> (w467:dbl[])
                    }
                    frame 2 {
                      n148 = Build Array (concatenate)(w474, w473) -> (w472:dbl[])
                    }
                  }
                  n149 = case shown="1" w431 {
                    tunnel: w434 -> [w450 w455 w460]
                    tunnel: w430 -> [w449 w453 w458]
                    tunnel: [w448 w455 w460] -> w433
                    tunnel: [w447 w452 w456] -> w432
                    tunnel: w435 -> [w447 w454 w456]
                    tunnel: [w446 w451 w457] -> w436
                    tunnel: w437 -> [w446 w451 w459]
                    frame 0, Default {
                      n150 = Build Array (concatenate)(w450, w449) -> (w448:dbl[])
                    }
                    frame 1 {
                      n151 = Build Array (concatenate)(w454, w453) -> (w452:dbl[])
                    }
                    frame 2 {
                      n152 = Build Array (concatenate)(w459, w458) -> (w457:dbl[])
                    }
                  }
                  n153 = Index Array(array=w430) -> (element #1=w444:dbl, element #2=w429:dbl)  [unwired: 2 in]
                  n154 = Subtract(x=w444, y=w429) -> (x-y=w445:dbl)
                }
                n155 = Less?(x=w421, y=1.5) -> (x < y?=w420:bool[])
                n156 = Boolean To (0,1)(Boolean=w420) -> (0, 1=w419:i16[])
                n157 = Add Array Elements(numeric array=w419) -> (sum=w418:i16)
                n158 = Greater?(x=w418, y=i16 1) -> (0:w416:bool)
              }
              n159 = call "Analyse_string_array.vi"("String array"=w384) -> ("Unique strings"=w380:string[])  [unwired: 1 in, 1 out]
              n160 = Array Max & Min(array=w390) -> (max value=w395:dbl, min value=w396:dbl)  [unwired: 2 out]
              n161 = Array Max & Min(array=w389) -> (max value=w394:dbl, min value=w393:dbl)  [unwired: 2 out]
              n162 = Array Max & Min(array=w388) -> (max value=w391:dbl, min value=w392:dbl)  [unwired: 2 out]
              n163 = Concatenate Strings(w380) -> (w379:string)
              n164 = Empty Array?(array=w380) -> (empty?=w378:bool)
              n165 = Build Array(w395, w396) -> (w387:dbl[])
              n166 = Build Array(w394, w393) -> (w385:dbl[])
              n167 = Build Array(w391, w392) -> (w386:dbl[])
              n168 = Empty String/Path?(string/path=w379) -> (empty?=w376:bool)
              n169 = Or(x=w378, y=w376) -> (x .or. y?=w377:bool)
              n170 = case shown="False" w377 {
                tunnel: w380 -> [_ w407]
                tunnel: ["" w406] -> w383
                frame True {
                }
                frame False {
                  n171 = Index Array(array=w407) -> (element=w406:string)  [unwired: 1 in]
                }
              }
            }
            "X per Figure" <- w361
            "Y per Figure" <- w359
            "Z per Figure" <- w360
            n172 = Array Max & Min(array=w373) -> (max value=w372:dbl, min value=w370:dbl)  [unwired: 2 out]
            n173 = Array Max & Min(array=w363) -> (max value=w368:dbl, min value=w369:dbl)  [unwired: 2 out]
            n174 = Array Max & Min(array=w362) -> (max value=w367:dbl, min value=w366:dbl)  [unwired: 2 out]
            n175 = Build Array(w372, w370) -> (→"All X":dbl[])
            n176 = Build Array(w368, w369) -> (→"All Y":dbl[])
            n177 = Build Array(w367, w366) -> (→"All Z":dbl[])
          }
          frame #5 {
            n178 = Or Array Elements(Boolean array=w478) -> (logical OR=w477:bool)
            n179 = case shown="True" w477 {
              tunnel: [TRUE ("Top Level") FALSE ("Top Level")] -> w476
              frame False {
              }
              frame True {
                n180 = One Button Dialog(message="Please select plains for the 2D plotter") -> ()  [unwired: 1 in, 1 out]
              }
            }
          }
          frame #6 {
            n181 = Build Path(base path=w484, name or relative path="Geometry") -> (appended path=w492:path)
            n182 = List Folder(path=w492) -> (filenames=w494:string[])  [unwired: 3 in, 3 out]
            n183 = local read "Manual_stl file"() -> (w490:bool)
            n184 = Build Array (concatenate)("", w494) -> (w493:string[])
            n185 = Index Array(array=w493, index="Stl File") -> (element=w488:string)
            n186 = case shown="False" w490 {
              tunnel: [w500 w504] -> w487
              tunnel: w488 -> [_ w505]
              tunnel: w483 -> [w499 _]
              frame False {
                n187 = for {
                  tunnel: w499 -> [w503] mode=indexing
                  tunnel: [w501] -> w500 mode=indexing
                  n188 = Concatenate Strings(w503, ".stl" ("string")) -> (w501:string)
                }
              }
              frame True {
                n189 = Build Array(w505) -> (w504:string[])
              }
            }
            n190 = property on="Stl File" class="Ring (strict)"("Strings []"=w493) -> ()  [unwired: 2 in, 2 out]
            n191 = for {
              tunnel: w492 -> [w498]
              tunnel: [w497] -> w489 mode=indexing
              tunnel: w487 -> [w496] mode=indexing
              n192 = Build Path(base path=w498, name or relative path=w496) -> (appended path=w497:path)
            }
            n193 = call "Get STL dimensions.vi"("Stl Filenames"=w489) -> ("Limits"=→"stl Limits":sgl[][], "stl Files"=→"stl Files":string[])  [unwired: 1 out]
          }
        }
      }
      frame "Create Input file" {
        n194 = local read "Plot"() -> (w511:i32[][])
        n195 = local read "Last Plot Index"() -> (w506:i32[])
        n196 = Index Array(array=w514, index (col)=1 ("disabled index (col)")) -> (element=w512:string[])  [unwired: 1 in]
        n197 = Index Array(array=w514, index (col)=0 ("disabled index (col)")) -> (element=w509:string[])  [unwired: 1 in]
        n198 = for {
          tunnel: w512 -> [w525]
          tunnel: w511 -> [w524] mode=indexing
          tunnel: [w523] -> w510 mode=concatenating
          tunnel: w509 -> [w522]
          tunnel: w507 -> [w521]
          tunnel: w506 -> [w518] mode=indexing
          i -> [w519]
          n199 = Increment(x=w519) -> (x+1=w520:i32)
          n200 = for {
            tunnel: [w535] -> w523 mode=indexing if=w537
            tunnel: w522 -> [w536]
            tunnel: w525 -> [w534]
            tunnel: w524 -> [w532] mode=indexing
            tunnel: w521 -> [w531]
            tunnel: w520 -> [w530]
            tunnel: w519 -> [w529]
            tunnel: w518 -> [w528]
            i -> [w527]
            n201 = Greater Or Equal To 0?(x=w532) -> (x >= 0?=w537:bool)
            n202 = Equal?(x=w527, y=w528) -> (x = y?=w526:bool)
            n203 = Number To Decimal String(number=w530) -> (decimal integer string=w533:string)  [unwired: 1 in]
            n204 = for {
              tunnel: w536 -> [w547] mode=indexing
              tunnel: [w546] -> w535 mode=indexing
              tunnel: w534 -> [w545] mode=indexing
              tunnel: w533 -> [w544]
              tunnel: w527 -> [w543]
              tunnel: w532 -> [w542]
              tunnel: w531 -> [w541]
              tunnel: w529 -> [w540]
              tunnel: w526 -> [w539]
              n205 = case shown="\"fAxisLabelZloc\"" w547 {
                tunnel: [w549 w554 w558 w561 "cScatterPointSize" w566 w573 w580 w637 w643 w648 w651 w657 w658 w672 w686 w702 w741 w785 w825 "0;0" w829 w833 w837 w841 w845 "0;0" w850 w852 "fvectorRotation" w860 w869 w885 w888 w892 w896 w900 w909 w913 w917 w921 w925 w929 w932 w939 w941 w943 w945 "MainTitleFontSize" "Font Size" w950 w956 w959 w963 w969 w973 w977 w981 w985 w990 w995 w1000 w1003 w1005] -> w546
                tunnel: w545 -> [_ _ _ _ _ _ _ _ _ _ _ _ _ _ _ _ _ _ _ _ _ _ _ _ _ _ _ _ _ _ _ _ _ _ _ _ _ _ _ _ _ _ _ _ _ _ _ _ _ _ _ _ _ _ _ _ _ _ _ _ _ _ _ w1005]
                tunnel: w544 -> [_ _ _ _ _ _ _ _ _ _ _ _ _ _ _ _ _ _ _ w825 _ _ _ _ _ _ _ _ _ _ _ _ _ _ _ _ _ _ _ _ _ _ _ _ _ _ _ _ _ _ _ _ _ _ _ _ _ _ _ _ _ _ _ _]
                tunnel: w543 -> [_ _ _ _ _ _ _ _ _ _ _ _ _ _ _ _ w705 w746 w789 _ _ _ _ _ _ _ _ _ _ _ _ _ _ _ _ _ _ _ _ _ _ _ _ _ _ _ _ _ _ _ _ _ _ _ _ _ _ _ _ _ _ _ _ _]
                tunnel: w542 -> [_ _ _ _ _ _ _ _ _ _ _ _ _ _ _ _ _ _ _ _ _ _ _ _ _ _ _ _ _ _ _ _ _ _ _ _ _ _ _ _ _ _ _ _ _ _ _ _ _ _ _ _ _ _ _ _ _ _ _ _ _ _ _ _]
                tunnel: w541 -> [_ _ _ _ _ _ _ _ _ _ _ _ _ _ _ _ _ _ _ _ _ _ _ _ _ _ _ _ _ _ _ _ _ _ _ _ _ _ _ _ _ _ _ _ _ _ _ _ _ _ _ _ _ _ _ _ _ _ _ _ _ _ _ _]
                tunnel: w540 -> [_ _ _ _ _ w565 _ w579 _ _ _ _ _ _ _ _ w704 w745 w788 _ _ _ _ _ _ _ _ _ w854 _ _ _ w875 _ _ _ _ w904 _ _ _ _ _ w935 _ _ _ _ _ _ _ _ _ _ _ _ _ _ _ _ _ _ _ _]
                tunnel: w539 -> [w548 w553 w557 w560 _ w570 w575 w583 w636 w642 w647 w650 w656 w662 w676 w690 w703 w744 w787 _ _ w828 w832 w836 w840 w844 _ w849 w856 _ w862 w871 w881 w887 w891 w895 w899 w908 w914 w916 w920 w924 w928 w931 w937 _ _ _ _ _ _ _ _ _ w968 w971 w975 w980 w984 w989 w994 w998 w1002 _]
                tunnel: "" -> [_ w552 w556 _ _ w568 w572 w582 w635 w641 w646 _ _ w660 w674 w689 w700 w743 w786 _ _ w827 w831 w835 w839 w843 _ w848 w855 _ _ _ _ w886 w890 w894 w898 _ w912 w915 w919 w923 w927 _ _ _ _ _ _ _ _ _ _ _ w967 _ _ w979 w983 _ w993 _ w1001 _]
                frame "cContourAct" {
                  n206 = Select(t="1", s=w548, f="0") -> (s? t:f=w549:string)
                }
                frame "cIncludeMin" {
                  n207 = Select(t="1", s=w553, f=w552) -> (s? t:f=w554:string)
                }
                frame "cLevNr" {
                  n208 = Select(t="20", s=w557, f=w556) -> (s? t:f=w558:string)
                }
                frame "cScatterAct" {
                  n209 = Select(t="1", s=w560, f="0") -> (s? t:f=w561:string)
                }
                frame "cScatterPointSize" {
                }
                frame "cdColorbarLabel" {
                  n210 = global read "Results_plotter_Global.vi" "Legend of ch names"() -> (w571:string[])
                  n211 = Index Array(array=w571, index=w565) -> (element=w569:string)
                  n212 = Select(t=w569, s=w570, f=w568) -> (s? t:f=w567:string)
                  n213 = call "TypesetInsideMathmode.vi"("DirtyString"=w567) -> ("Mathmode String"=w566:string)  [unwired: 8 in, 2 out]
                }
                frame "cdColorbarLogarithmic" {
                  n214 = case shown="\"Lin\"" "Plotting" {
                    tunnel: ["0" ("fAxisLimY Location") "1" ("fAxisLimY Location")] -> w574
                    frame "Lin" {
                    }
                    frame "Log" {
                    }
                  }
                  n215 = Select(t=w574, s=w575, f=w572) -> (s? t:f=w573:string)
                }
                frame "cdColorbarRange" {
                  n216 = local read "C Limits"() -> (w593:cluster{dbl[]}[])
                  n217 = local read "mSingleColorbar"() -> (w587:bool)
                  n218 = case shown="True" w587 {
                    tunnel: w593 -> [w618 w620]
                    tunnel: [w615 w619] -> w588
                    tunnel: w579 -> [w617 _]
                    frame False {
                      n219 = Index Array(array=w618, index=w617) -> (element=w616:cluster{dbl[]})
                      n220 = Unbundle(w616) -> (w615:dbl[])
                    }
                    frame True {
                      n221 = for {
                        tunnel: [w621] -> w619 mode=concatenating
                        tunnel: w620 -> [w622] mode=indexing
                        n222 = Unbundle(w622) -> (w621:dbl[])
                      }
                    }
                  }
                  n223 = local read "Concentration?"() -> (w584:bool)
                  n224 = case shown="True" w584 {
                    tunnel: [w598 w604] -> w590
                    tunnel: [w594 w603] -> w589
                    tunnel: w588 -> [w601 w602]
                    frame False {
                      n225 = Array Max & Min(array=w601) -> (max value=w596:dbl, min value=w597:dbl)  [unwired: 2 out]
                      n226 = Subtract(x=w596, y=w597) -> (x-y=w600:dbl)
                      n227 = Multiply(x=0.05, y=w600) -> (x*y=w595:dbl)
                      n228 = Subtract(x=w597, y=w595) -> (x-y=w598:dbl)
                      n229 = Add(x=w596, y=w595) -> (x+y=w594:dbl)
                    }
                    frame True {
                      n230 = call <vilib>:"Std Deviation and Variance.vi"("X"=w602) -> ("mean"=w606:dbl, "standard deviation"=w607:dbl)  [unwired: 1 in, 1 out]
                      n231 = Multiply(x=w607, y=4.0) -> (x*y=w609:dbl)
                      n232 = Multiply(x=w607, y=6.0) -> (x*y=w605:dbl)
                      n233 = Subtract(x=w606, y=w605) -> (x-y=w604:dbl)
                      n234 = Add(x=w606, y=w609) -> (x+y=w603:dbl)
                    }
                  }
                  n235 = local read "Plotting"() -> (w592:enum8{"Lin", "Log"})
                  n236 = case shown="\"Lin\"" w592 {
                    tunnel: [w623 w626] -> w591
                    tunnel: w590 -> [w623 _]
                    tunnel: w589 -> [_ w627]
                    tunnel: "No Of decades" -> [_ w625]
                    frame "Lin" {
                    }
                    frame "Log" {
                      n237 = case shown="6" w625 {
                        tunnel: [100.0 1000.0 10000.0 100000.0 1000000.0 10000000.0 10.0] -> w624
                        frame 2 {
                        }
                        frame 3 {
                        }
                        frame 4 {
                        }
                        frame 5 {
                        }
                        frame 6 {
                        }
                        frame 7, Default {
                        }
                        frame 1 {
                        }
                      }
                      n238 = Divide(x=w627, y=w624) -> (x/y=w626:dbl)
                    }
                  }
                  n239 = case shown="True" "Range Auto" {
                    tunnel: w591 -> [_ w614]
                    tunnel: w589 -> [_ w613]
                    tunnel: ["cdColorbarRange" w612] -> w581
                    frame False {
                    }
                    frame True {
                      n240 = call "Non equal Min Max.vi"("Max"=w613, "Min"=w614) -> ("Limits"=w612:string)  [unwired: 1 in]
                      n241 = local write "cdColorbarRange"(w612) -> ()
                    }
                  }
                  n242 = Select(t=w581, s=w583, f=w582) -> (s? t:f=w580:string)
                }
                frame "cdColormap" {
                  n243 = Select(t="jet", s=w636, f=w635) -> (s? t:f=w637:string)
                }
                frame "cdMethodInterp" {
                  n244 = local read "Plotting"() -> (w639:enum8{"Lin", "Log"})
                  n245 = case shown="\"Log\"" w639 {
                    tunnel: ["cubic" "Natural"] -> w640
                    frame "Lin" {
                    }
                    frame "Log" {
                    }
                  }
                  n246 = Select(t=w640, s=w642, f=w641) -> (s? t:f=w643:string)
                }
                frame "cdSpaceInterp" {
                  n247 = Select(t="1", s=w647, f=w646) -> (s? t:f=w648:string)
                }
                frame "d3DAct", "lLocationAct" {
                  n248 = Select(t="1", s=w650, f="0") -> (s? t:f=w651:string)
                }
                frame "dContourTransparency" {
                  n249 = Select(t="Transparency", s=w656, f="") -> (s? t:f=w657:string)
                }
                frame "fAxisLabelX" {
                  n250 = global read "Results_plotter_Global.vi" "3D Ch Names"() -> (w671:string[])
                  n251 = Index Array(array=w671, index=0) -> (element=w664:string)
                  n252 = call "Fast_string_Replace.vi"("Replace match with:"=" ", "Input String"=w664, "matchThis"=":" ("regular expression")) -> ("Output String"=w668:string)  [unwired: 1 in, 1 out]
                  n253 = call "Fast_string_Replace.vi"("Replace match with:"=" ", "Input String"=w668, "matchThis"="  " ("regular expression")) -> ("Output String"=w667:string)  [unwired: 1 in, 1 out]
                  n254 = call <vilib>:"Trim Whitespace.vi"("string"=w667) -> ("trimmed string"=w661:string)  [unwired: 1 in]
                  n255 = Select(t=w661, s=w662, f=w660) -> (s? t:f=w659:string)
                  n256 = call "TypesetInsideMathmode.vi"("DirtyString"=w659) -> ("Mathmode String"=w658:string)  [unwired: 8 in, 2 out]
                }
                frame "fAxisLabelY" {
                  n257 = global read "Results_plotter_Global.vi" "3D Ch Names"() -> (w685:string[])
                  n258 = Index Array(array=w685, index=1) -> (element=w678:string)
                  n259 = call "Fast_string_Replace.vi"("Replace match with:"=" ", "Input String"=w678, "matchThis"=":" ("regular expression")) -> ("Output String"=w682:string)  [unwired: 1 in, 1 out]
                  n260 = call "Fast_string_Replace.vi"("Replace match with:"=" ", "Input String"=w682, "matchThis"="  " ("regular expression")) -> ("Output String"=w681:string)  [unwired: 1 in, 1 out]
                  n261 = call <vilib>:"Trim Whitespace.vi"("string"=w681) -> ("trimmed string"=w675:string)  [unwired: 1 in]
                  n262 = Select(t=w675, s=w676, f=w674) -> (s? t:f=w673:string)
                  n263 = call "TypesetInsideMathmode.vi"("DirtyString"=w673) -> ("Mathmode String"=w672:string)  [unwired: 8 in, 2 out]
                }
                frame "fAxisLabelZloc" {
                  n264 = global read "Results_plotter_Global.vi" "3D Ch Names"() -> (w699:string[])
                  n265 = Index Array(array=w699, index=2) -> (element=w692:string)
                  n266 = call "Fast_string_Replace.vi"("Replace match with:"=" ", "Input String"=w692, "matchThis"=":" ("regular expression")) -> ("Output String"=w696:string)  [unwired: 1 in, 1 out]
                  n267 = call "Fast_string_Replace.vi"("Replace match with:"=" ", "Input String"=w696, "matchThis"="  " ("regular expression")) -> ("Output String"=w695:string)  [unwired: 1 in, 1 out]
                  n268 = call <vilib>:"Trim Whitespace.vi"("string"=w695) -> ("trimmed string"=w688:string)  [unwired: 1 in]
                  n269 = Select(t=w688, s=w690, f=w689) -> (s? t:f=w687:string)
                  n270 = call "TypesetInsideMathmode.vi"("DirtyString"=w687) -> ("Mathmode String"=w686:string)  [unwired: 8 in, 2 out]
                }
                frame "fAxisLimX" {
                  n271 = case shown="True" "X Limits Auto" {
                    tunnel: ["Location X limits" w708] -> w701
                    tunnel: w705 -> [_ _]
                    tunnel: w704 -> [_ w713]
                    frame False {
                    }
                    frame True {
                      n272 = local read "stl Limits"() -> (w711:sgl[][])
                      n273 = case shown="True" "Same Location limits for all plots" {
                        tunnel: [w722 w734] -> w710
                        tunnel: [w721 w733] -> w709
                        tunnel: w713 -> [w719 _]
                        tunnel: "Show whole Stl file" -> [w715 w732]
                        tunnel: w711 -> [w718 w731]
                        frame False {
                          n274 = local read "X per Figure"() -> (w720:dbl[][])
                          n275 = Index Array(array=w720, index (row)=w719) -> (element=w717:dbl[])  [unwired: 1 in]
                          n276 = case shown="True" w715 {
                            tunnel: w718 -> [_ w726]
                            tunnel: w717 -> [w723 w725]
                            tunnel: [w723 w724] -> w716
                            frame False {
                            }
                            frame True {
                              n277 = Index Array(array=w726, index (row)=0) -> (element=w727:sgl[])  [unwired: 1 in]
                              n278 = Build Array (concatenate)(w725, w727) -> (w724:dbl[])
                            }
                          }
                          n279 = Index Array(array=w716) -> (element #1=w722:dbl, element #2=w721:dbl)  [unwired: 2 in]
                        }
                        frame True {
                          n280 = local read "All X"() -> (w730:dbl[])
                          n281 = case shown="True" w732 {
                            tunnel: w731 -> [_ w739]
                            tunnel: w730 -> [w735 w737]
                            tunnel: [w735 w736] -> w729
                            frame False {
                            }
                            frame True {
                              n282 = Index Array(array=w739, index (row)=0) -> (element=w738:sgl[])  [unwired: 1 in]
                              n283 = Build Array (concatenate)(w737, w738) -> (w736:dbl[])
                            }
                          }
                          n284 = Array Max & Min(array=w729) -> (max value=w734:dbl, min value=w733:dbl)  [unwired: 2 out]
                        }
                      }
                      n285 = call "Set Plot limits.vi"("Min"=w709, "Max"=w710) -> ("resulting string"=w708:string)
                    }
                  }
                  "X Limit" <- w701
                  n286 = Select(t=w701, s=w703, f=w700) -> (s? t:f=w702:string)
                }
                frame "fAxisLimY" {
                  n287 = case shown="True" "Y Limits Auto" {
                    tunnel: ["Location Y limits" w749] -> w742
                    tunnel: w746 -> [_ w755]
                    tunnel: w745 -> [_ w754]
                    frame False {
                    }
                    frame True {
                      n288 = local read "Show whole Stl file"() -> (w753:bool)
                      n289 = local read "stl Limits"() -> (w752:sgl[][])
                      n290 = local read "Same Location limits for all plots"() -> (w756:bool)
                      n291 = case shown="False" w756 {
                        tunnel: [w764 w776] -> w751
                        tunnel: [w763 w775] -> w750
                        tunnel: w755 -> [_ _]
                        tunnel: w754 -> [w761 _]
                        tunnel: w753 -> [w759 w772]
                        tunnel: w752 -> [w760 w771]
                        frame False {
                          n292 = local read "Y per Figure"() -> (w762:dbl[][])
                          n293 = Index Array(array=w762, index (row)=w761) -> (element=w758:dbl[])  [unwired: 1 in]
                          n294 = case shown="True" w759 {
                            tunnel: w758 -> [w765 w768]
                            tunnel: [w765 w767] -> w757
                            tunnel: w760 -> [_ w766]
                            frame False {
                            }
                            frame True {
                              n295 = Index Array(array=w766, index (row)=1) -> (element=w769:sgl[])  [unwired: 1 in]
                              n296 = Build Array (concatenate)(w768, w769) -> (w767:dbl[])
                            }
                          }
                          n297 = Index Array(array=w757) -> (element #1=w764:dbl, element #2=w763:dbl)  [unwired: 2 in]
                        }
                        frame True {
                          n298 = local read "All Y"() -> (w774:dbl[])
                          n299 = case shown="False" w772 {
                            tunnel: w774 -> [w777 w780]
                            tunnel: [w777 w779] -> w773
                            tunnel: w771 -> [_ w778]
                            frame False {
                            }
                            frame True {
                              n300 = Index Array(array=w778, index (row)=1) -> (element=w781:sgl[])  [unwired: 1 in]
                              n301 = Build Array (concatenate)(w780, w781) -> (w779:dbl[])
                            }
                          }
                          n302 = Array Max & Min(array=w773) -> (max value=w776:dbl, min value=w775:dbl)  [unwired: 2 out]
                        }
                      }
                      n303 = call "Set Plot limits.vi"("Min"=w750, "Max"=w751) -> ("resulting string"=w749:string)
                    }
                  }
                  "Y Limit" <- w742
                  n304 = Select(t=w742, s=w744, f=w743) -> (s? t:f=w741:string)
                }
                frame "fAxisLimZloc" {
                  (unwired) FALSE
                  n305 = case shown="True" "Z Limits Auto" {
                    tunnel: ["Location Z limits" w791] -> w783
                    tunnel: w789 -> [_ w797]
                    tunnel: w788 -> [_ w796]
                    frame False {
                    }
                    frame True {
                      n306 = local read "Show whole Stl file"() -> (w795:bool)
                      n307 = local read "stl Limits"() -> (w794:sgl[][])
                      n308 = local read "Same Location limits for all plots"() -> (w798:bool)
                      n309 = case shown="True" w798 {
                        tunnel: [w806 w818] -> w793
                        tunnel: [w805 w817] -> w792
                        tunnel: w797 -> [_ _]
                        tunnel: w796 -> [w803 _]
                        tunnel: w795 -> [w801 w814]
                        tunnel: w794 -> [w802 w813]
                        frame False {
                          n310 = local read "Z per Figure"() -> (w804:dbl[][])
                          n311 = Index Array(array=w804, index (row)=w803) -> (element=w800:dbl[])  [unwired: 1 in]
                          n312 = case shown="False" w801 {
                            tunnel: w800 -> [w807 w810]
                            tunnel: [w807 w809] -> w799
                            tunnel: w802 -> [_ w808]
                            frame False {
                            }
                            frame True {
                              n313 = Index Array(array=w808, index (row)=2) -> (element=w811:sgl[])  [unwired: 1 in]
                              n314 = Build Array (concatenate)(w810, w811) -> (w809:dbl[])
                            }
                          }
                          n315 = Index Array(array=w799) -> (element #1=w806:dbl, element #2=w805:dbl)  [unwired: 2 in]
                        }
                        frame True {
                          n316 = local read "All Z"() -> (w816:dbl[])
                          n317 = case shown="True" w814 {
                            tunnel: w816 -> [w819 w822]
                            tunnel: [w819 w821] -> w815
                            tunnel: w813 -> [_ w820]
                            frame False {
                            }
                            frame True {
                              n318 = Index Array(array=w820, index (row)=2) -> (element=w823:sgl[])  [unwired: 1 in]
                              n319 = Build Array (concatenate)(w822, w823) -> (w821:dbl[])
                            }
                          }
                          n320 = Array Max & Min(array=w815) -> (max value=w818:dbl, min value=w817:dbl)  [unwired: 2 out]
                        }
                      }
                      n321 = call "Set Plot limits.vi"("Min"=w792, "Max"=w793) -> ("resulting string"=w791:string)
                    }
                  }
                  "Z Limit" <- w783
                  n322 = Select(t=w783, s=w787, f=w786) -> (s? t:f=w785:string)
                }
                frame "fFigureNr" {
                }
                frame "fFlipNormal" {
                }
                frame "fFontSize" {
                  n323 = Select(t="10", s=w828, f=w827) -> (s? t:f=w829:string)
                }
                frame "fGrid" {
                  n324 = Select(t="1;1;1", s=w832, f=w831) -> (s? t:f=w833:string)
                }
                frame "fGridMinor" {
                  n325 = Select(t="0;0;0", s=w836, f=w835) -> (s? t:f=w837:string)
                }
                frame "fInterpreterText" {
                  n326 = Select(t="latex", s=w840, f=w839) -> (s? t:f=w841:string)
                }
                frame "fLogAxis" {
                  n327 = Select(t="0;0;0", s=w844, f=w843) -> (s? t:f=w845:string)
                }
                frame "fReverseAxis" {
                }
                frame "fTickLabel" {
                  n328 = Select(t="1;1;1", s=w849, f=w848) -> (s? t:f=w850:string)
                }
                frame "fTitle" {
                  n329 = local read "Plot Titles"() -> (w858:string[])
                  n330 = Index Array(array=w858, index=w854) -> (element=w857:string)
                  n331 = Select(t=w857, s=w856, f=w855) -> (s? t:f=w853:string)
                  n332 = call "TypesetInsideMathmode.vi"("DirtyString"=w853) -> ("Mathmode String"=w852:string)  [unwired: 8 in, 2 out]
                }
                frame "fVectorRotations" {
                }
                frame "fVectorComponentNr" {
                  n333 = local read "Streamlines"() -> (w864:bool)
                  n334 = local read "Vectors"() -> (w865:bool)
                  n335 = Or(x=w865, y=w864) -> (x .or. y?=w863:bool)
                  n336 = And(x=w863, y=w862) -> (x .and. y?=w861:bool)
                  n337 = Select(t="0", s=w861, f="3") -> (s? t:f=w860:string)
                }
                frame "vVectorAct" {
                  n338 = And(x="Vectors", y=w871) -> (x .and. y?=w870:bool)
                  n339 = Select(t="1", s=w870, f="0") -> (s? t:f=w869:string)
                }
                frame "gGeometryAct" {
                  n340 = local read "Manual_stl file"() -> (w876:bool)
                  n341 = Select(t=0, s=w876, f=w875) -> (s? t:f=w878:i32)
                  n342 = local read "stl Files"() -> (w879:string[])
                  n343 = Index Array(array=w879, index=w878) -> (element=w874:string)
                  n344 = Empty String/Path?(string/path=w874) -> (empty?=w880:bool)
                  n345 = Compound Arithmetic op=AND(invert w880, w881) -> (w882:bool)
                  n346 = Select(t="1", s=w882, f="0") -> (s? t:f=w885:string)
                }
                frame "gldEdgeColor" {
                  n347 = Select(t="k", s=w887, f=w886) -> (s? t:f=w888:string)
                }
                frame "gldEdgeTransparency" {
                  n348 = Select(t="1", s=w891, f=w890) -> (s? t:f=w892:string)
                }
                frame "gldFaceColor" {
                  n349 = Select(t="#acada9", s=w895, f=w894) -> (s? t:f=w896:string)
                }
                frame "gldFaceTransparency" {
                  n350 = Select(t="1", s=w899, f=w898) -> (s? t:f=w900:string)
                }
                frame "gldGeometryFilename" {
                  n351 = Select(t=0, s="Manual_stl file", f=w904) -> (s? t:f=w902:i32)
                  n352 = local read "stl Files"() -> (w907:string[])
                  n353 = Index Array(array=w907, index=w902) -> (element=w905:string)
                  n354 = Select(t=w905, s=w908, f="") -> (s? t:f=w909:string)
                }
                frame "gldGeometryRotations" {
                  n355 = Select(t="0;0;0" ("format string"), s=w914, f=w912) -> (s? t:f=w913:string)
                }
                frame "gldGeometryTranslations" {
                  n356 = Select(t="0;0;0", s=w916, f=w915) -> (s? t:f=w917:string)
                }
                frame "lMarkerColor" {
                  n357 = Select(t="r", s=w920, f=w919) -> (s? t:f=w921:string)
                }
                frame "lMarkerSize" {
                  n358 = Select(t="2", s=w924, f=w923) -> (s? t:f=w925:string)
                }
                frame "lMarkerType" {
                  n359 = Select(t="*", s=w928, f=w927) -> (s? t:f=w929:string)
                }
                frame "ldListDatafileShown" {
                  n360 = local read "ldListDatafileShown"() -> (w936:string[])
                  n361 = Index Array(array=w936, index=w935) -> (element=w933:string)
                  n362 = Select(t=w933, s=w931, f="") -> (s? t:f=w932:string)
                }
                frame "ldViewAngles" {
                  n363 = Select(t="ViewAngles", s=w937, f="") -> (s? t:f=w939:string)
                }
                frame "mGraphsxColumn" {
                  n364 = Number To Decimal String(number="nCols") -> (decimal integer string=w941:string)  [unwired: 1 in]
                }
                frame "mGraphsxRow" {
                  n365 = Number To Decimal String(number="nRows") -> (decimal integer string=w943:string)  [unwired: 1 in]
                }
                frame "mMainTitle" {
                  n366 = local read "Final Title"() -> (w946:string)
                  n367 = call "TypesetInsideMathmode.vi"("DirtyString"=w946) -> ("Mathmode String"=w945:string)  [unwired: 8 in, 2 out]
                }
                frame "mMainTitleFontSize" {
                }
                frame "mFontSize" {
                }
                frame "mSingleColorbarLocation" {
                  n368 = Format Into String(format string="%s;%s;%s;%s", "LeftEdge", "BottomEdge", "Width", "Height") -> (resulting string=w950:string)  [unwired: 2 in, 1 out]
                }
                frame "mSingleColorbar" {
                  n369 = Select(t="1", s="mSingleColorbar", f="0") -> (s? t:f=w956:string)
                }
                frame "mSpaceX" {
                  n370 = local read "Same Location limits for all plots"() -> (w962:bool)
                  n371 = Select(t="0.2", s=w962, f="2.2") -> (s? t:f=w959:string)
                }
                frame "mSpaceY" {
                  n372 = local read "Same Location limits for all plots"() -> (w966:bool)
                  n373 = Select(t="2.5", s=w966, f="2.5") -> (s? t:f=w963:string)
                }
                frame "sBottomEdge" {
                  n374 = Select(t="4.85", s=w968, f=w967) -> (s? t:f=w969:string)
                }
                frame "sFigRenderer" {
                  n375 = Select(t="opengl", s=w971, f="") -> (s? t:f=w973:string)
                }
                frame "sFormatFig" {
                  n376 = Select(t="pdf", s=w975, f="") -> (s? t:f=w977:string)
                }
                frame "sLeftEdge" {
                  n377 = Select(t="0.5", s=w980, f=w979) -> (s? t:f=w981:string)
                }
                frame "sPlotHeight", "sPlotWidth" {
                  n378 = Select(t="20", s=w984, f=w983) -> (s? t:f=w985:string)
                }
                frame "tStreamlineAct" {
                  n379 = And(x="Streamlines", y=w989) -> (x .and. y?=w988:bool)
                  n380 = Select(t="1", s=w988, f="0") -> (s? t:f=w990:string)
                }
                frame "tStreamlineColor" {
                  n381 = Select(t="k", s=w994, f=w993) -> (s? t:f=w995:string)
                }
                frame "tStreamlineDensity" {
                  n382 = Select(t="Streamline Density", s=w998, f="") -> (s? t:f=w1000:string)
                }
                frame "tStreamlineWidth" {
                  n383 = Select(t="1", s=w1002, f=w1001) -> (s? t:f=w1003:string)
                }
                frame Default {
                }
              }
            }
          }
        }
        n384 = Build Array (concatenate)(w509, w510) -> (→"Table":string[][])
      }
      frame "Save Input File" {
        # "Create matching output directory, as MATLAB won't, and it may not exist, if running from EXE"
        n385 = local read "U Vector"() -> (w1023:u16)
        n386 = local read "W Vector"() -> (w1021:u16)
        n387 = local read "V Vector"() -> (w1022:u16)
        n388 = local read "Selectors"() -> (w1019:i32[])
        n389 = Build Array(w1023, w1022, w1021) -> (w1020:u16[])
        n390 = local read "Table"() -> (w1024:string[][])
        n391 = for {
          tunnel: w1020 -> [w1032] mode=indexing
          tunnel: w1019 -> [w1036] mode=indexing
          tunnel: w1017 -> [w1035]
          tunnel: w1016 -> [w1033]
          tunnel: [w1032] -> w1015 mode=indexing
          tunnel: w1014 -> [w1031] mode=indexing
          n392 = Equal?(x=w1032, y=w1036) -> (x = y?=w1034:bool)
          n393 = case shown="False" w1034 {
            tunnel: w1035 -> [w1042 _]
            tunnel: w1032 -> [w1041 _]
            tunnel: w1033 -> [w1040 _]
            tunnel: w1031 -> [w1037 _]
            frame False {
              n394 = Index Array(array=w1040, index=w1041) -> (element=w1039:string)
              n395 = call "Read_Write_Template.vi"("Template File"=w1042, "Mode"=Global_mode."Write Global to File", "Single Value In"=w1039, "Data type"=w1037) -> ()  [unwired: 4 in, 8 out]
            }
            frame True {
            }
          }
        }
        n396 = Build Path(base path=w1018, name or relative path="Input2D.xls") -> (appended path=w1027:path)
        n397 = Array To Spreadsheet String(array=w1024, 3:"%s" ("format string")) -> (spreadsheet string=w1028:string)  [unwired: 1 in]
        n398 = Write to Text File(file (use dialog)=w1027, text=w1028) -> (refnum out=w1010:refnum<file>, error out=w1011:errorcluster)  [unwired: 2 in, 1 out]
        n399 = Close File(refnum=w1010, error in=w1011) -> (error out=w1009:errorcluster)  [unwired: 1 out]
        n400 = Build Path(base path=w1008, name or relative path="Output") -> (appended path=w1013:path)
        n401 = Build Path(base path=w1013, name or relative path=w1007) -> (appended path=w1006:path)
        n402 = call <vilib>:"Create Directory Recursive.vi"("error in (no error)"=w1009, "directory"=w1006) -> ()  [unwired: 3 in, 3 out]
        n403 = local write "Selectors"(w1015) -> ()
      }
      frame "Run MATLAB Code" {
        n404 = call "Call_MATLAB_Suite.vi"("Mode"=MATLAB_Mode."2D Plotter") -> ("Output file"=→"Output file":path, "error out"=w1043:errorcluster)  [unwired: 2 in, 1 out]
        n405 = case shown="Error .." w1043 {
          selector: w1043 -> [_ w1053]
          tunnel: [TRUE ("Top Level") FALSE ("Top Level")] -> w1049
          frame No Error {
          }
          frame Error {
            n406 = Unbundle By Name(w1053) -> ("source"=w1052:string)
            n407 = One Button Dialog(message=w1052) -> ()  [unwired: 1 in, 1 out]
          }
        }
        n408 = Select(t="Display PDF with save option", s="Show Save Option?", f="Display PDF" ("t")) -> (s? t:f=w1044:string)
      }
      frame "Display PDF" {
        n409 = local read "Output file"() -> (w1055:path)
        n410 = call "Open PDF in desired reader.vi"("Path"=w1055) -> ()  [unwired: 2 in, 1 out]
      }
      frame "Display PDF with save option" {
        n411 = local read "Plot Folder"() -> (w1058:string[])
        n412 = local read "Output file"() -> (w1061:path)
        n413 = stacked-sequence {
          tunnel: w1061 -> [w1065 w1071]
          tunnel: w1058 -> [w1062 _]
          frame #0 {
            n414 = call "Display PDF File for Preview.vi"("Data Directories"=w1062, "PDF file"=w1065) -> ("Filename Out"=w1064:string)  [unwired: 8 in, 1 out]
            n415 = Empty String/Path?(string/path=w1064) -> (empty?=w1063:bool)
            n416 = case shown="False" w1063 {
              tunnel: w1065 -> [w1068 _]
              tunnel: w1064 -> [w1067 _]
              tunnel: w1062 -> [w1066 _]
              frame False {
                n417 = local read "Duplicate Plot"() -> (w1069:bool)
                n418 = call "Save PDF files.vi"("Duplicate Plot"=w1069, "Open in Acrobat"="Open in Acrobat", "Desired Filename"=w1067, "Data Directories"=w1066, "PDF file in"=w1068) -> ()  [unwired: 5 in, 2 out]
              }
              frame True {
              }
            }
          }
          frame #1 {
            n419 = Delete(path (use dialog)=w1071) -> ()  [unwired: 4 in, 3 out]
          }
        }
      }
      frame "End" {
      }
    }
  }
  "AuditTrail" <- w21
  "Saved Automatically?" <- FALSE
